vi "Pick&Place_ladder_shih_v8_toolcenter.vi"() -> ()   [LabVIEW 2016]
uses:
  WTF is this.ctl
  Classes/Controllers/I-O/Copy of NI-DAQ Folder/NI-DAQ.lvclass
  D:/INTT/V1/Classes/Controllers/I-O/Copy of I-O Folder/I-O.lvclass
  Classes/Controllers/Dispenser/Copy of Ultimus V2 Folder/Ultimus V2.lvclass
  <vilib>/Analysis/coordinate.llb/2D Cartesian Coordinate Rotation (Scalar).vi
  <vilib>/Utility/file.llb/Read Delimited Spreadsheet (DBL).vi
  <vilib>/Utility/file.llb/Write Delimited Spreadsheet (DBL).vi
  Classes/Controllers/Motion/Copy of Motion Folder/Motion.lvclass
  Classes/Controllers/Camera/Copy of Controller Folder/Controller.lvclass
  <vilib>/Analysis/NI_AALPro.lvlib
  Classes/Controllers/I-O/Copy of I-O Folder/I-O.lvclass
panel:
  out "file indicator":dbl[][](array[numeric])
  out "?":dbl[](array[numeric]) format="%#_8g"
  in  "offset":dbl[](array[numeric])=[0.0, 0.0, 0.0, 0.0] format="%#_8g"
  out "HDI center positions":dbl[][](array[numeric]) format="%#_8g"
  out "HDI center positions":dbl[][](array[numeric])=[[459.92445114002015, 980.2358762511564, 78.77350133595746, 0.0015214873297426886]] format="%#_8g"
  out "CT sum up":dbl[](array[numeric])
  in  "txt switch":bool
  in  "MPT offset":dbl[][](array[numeric])=[[0.0, 0.0, 0.0, 0.0], [0.0, 0.0, 0.0, 0.0]] format="%#_8g"
  out "CT HPoS":dbl[][](array[numeric]) format="%#_8g"
  out "chip distance by OGP":dbl format="%#_8g"
  out "displacement":dbl[](array[numeric])
  out "gantry position test":dbl[](array[numeric])
  out "gantry target position":dbl[](array[numeric])
  out "chip distance by gantry":dbl format="%#_8g"
  out "after SL":dbl[](array[numeric]) format="%#_8g"
  out "after SR":dbl[](array[numeric]) format="%#_8g"
  out "after NL":dbl[](array[numeric]) format="%#_8g"
  out "S chip":dbl[](array[numeric]) format="%#_8g"
  out "N chip":dbl[](array[numeric]) format="%#_8g"
  in  "?":path=path "C:/Users/PAGANIS/Desktop/shih cheng wei/OGP/test1-2.txt"
  out "bless from OGP !!! Center of  stave":dbl[](array[numeric])
  out "bless from OGP !! measured stave size":dbl[](array[numeric])
  in  "Bless from OGP":bool
  out "FROM Detail !!! Center of module on stave":dbl[](array[numeric])
  out "FROM Detail !! measured stave size":dbl[](array[numeric])
  in  "Align Stave in detail":bool
  in  "check height?":bool
  in  "Uttimus presssure":i64=10
  out "Status":bool
  out "measured HDI top-left position":dbl[][](array[numeric])
  in  "HDI vacuum channel":i32=18
  in  "vacuum":bool=TRUE
  in  "HDI vacuum":bool
  out "measured stave size":dbl[](array[numeric])
  out "Stave mark":dbl[][](array[numeric])
  out "Center of module on stave":dbl[](array[numeric])
  out "Measured HDI size":dbl[][](array[numeric])
  out "MPT positions on stave":T1[][](array[typedef])
  in  "Default Stave dimension":dbl[](array[numeric])=[34.0, 472.0, -0.335295, -0.000320234]
  in  "Default Stave upper left mark":dbl[](array[numeric])=[584.376, 675.576, 70.9882, 0.000840064]
  out "Needle parking position":dbl[](array[numeric])
  in  "Uppler / Lower Stave":bool=TRUE
  out "Gantry current position":dbl[](array[numeric])
  in  "READ Position":bool
  in  "Needle Height Compenstation\n(glue gap)":dbl=0.33
  in  "Needle Alignment":bool
  in  "Parking position":dbl[](array[numeric])=[625.0, 625.0, 0.0, 0.01]
  in  "GOTO":bool
  in  "Default Pickup Tool Position":dbl[][](array[numeric])=[[152.226, 682.729, 36.8129, -0.0151898], [700.0, 800.0, 20.0, 0.01]]
  in  "deposit glue module":i32=1
  in  "Default HDI alignment \nmark position":dbl[](array[numeric])=[448.322, 976.582, 74.9872, 0.000191129]
  in  "Default HDI size":dbl[](array[numeric])=[24.2437, 231.446, -0.099339, 0.000191129]
  out "# of tasks excuted":i32
  out "PickupTool \nCenterPosition":dbl[](array[numeric]) format="%#_8g"
  in  "Inititalize":bool
  in  "Pick and place":bool
  in  "Deposit Glue":bool
  in  "Measure Pickup Tools":bool
  in  "Align Stave":bool
  out "default module position on stave":dbl[][](array[numeric])
  in  "Stop":bool
  in  "Measure HDI":bool
  # "Ladder Assembly"
  # "To switch the north/south\ntxt file \nswitch \noffset\nmodule pick up tool\nmodule direction"
  # "Upper\nmodule"
  # "Lower\nmodule"
  # "Sensor 0.32 -> 200 micron glue thickness\nChips 0.37-> 140 micron glue thickness"
  # "ACTIONS"
  # "theta had *-1"
  # "Pick up tool and needle"
  # "Module infomation"
  # "Pick and Place"
  # "CT"
  # "+"
  # "+"
  # "="
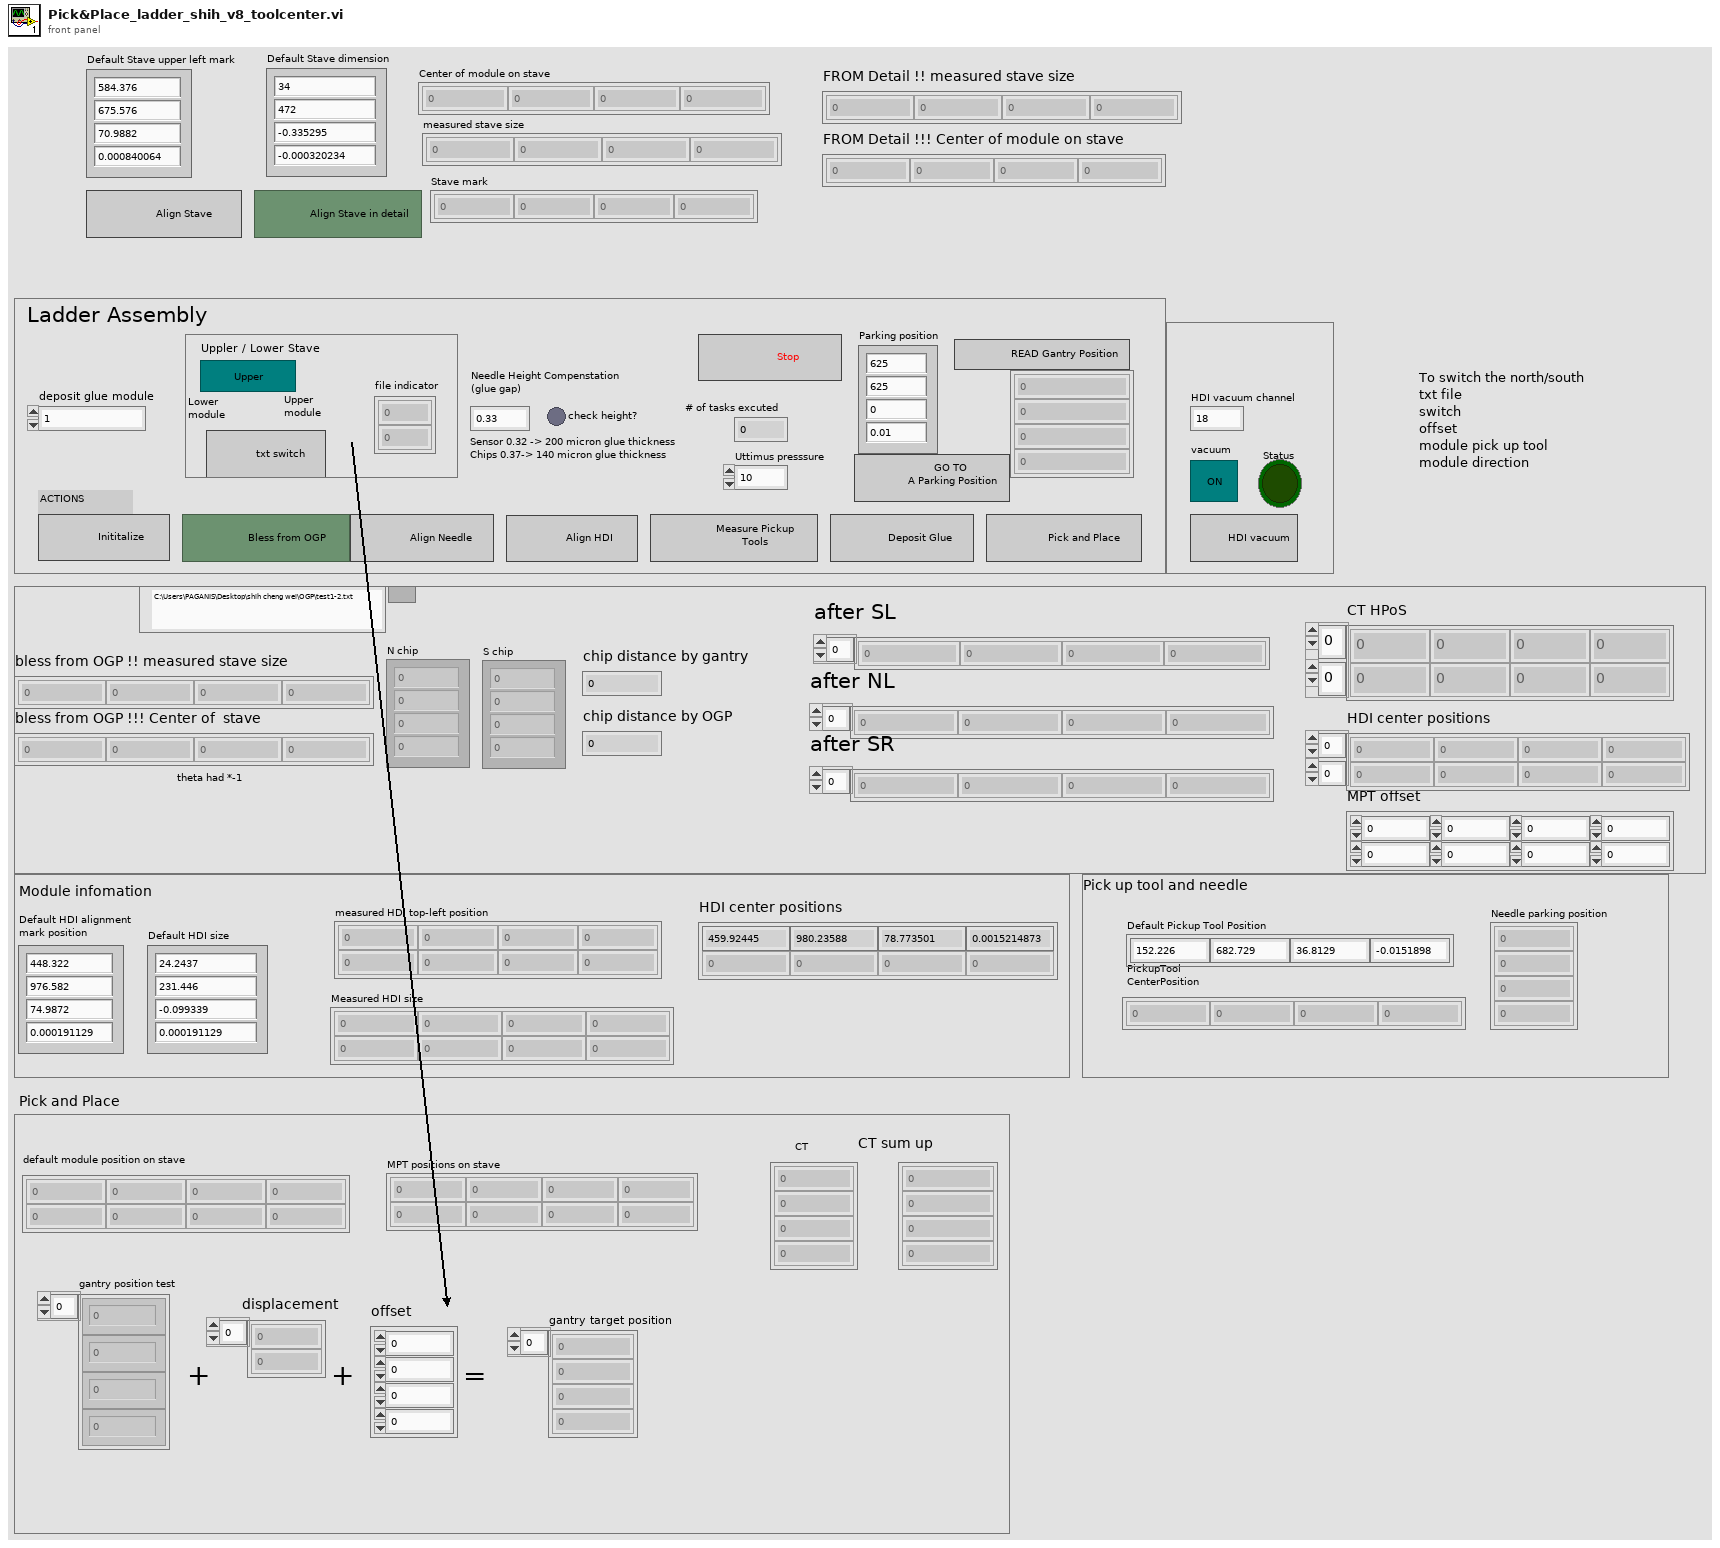
[diagram p1: front panel]
types:
  T1 = typedef "WTF is this.ctl" = dbl
  T2 = typedef "Controller.lvclass/Controllers.ctl" = cluster{"Copy of Motion.lvclass":refnum<class "Motion.lvclass">, "Copy of I-O.lvclass":refnum<class "I-O.lvclass">, "Copy of Dispenser.lvclass":refnum<class "Dispenser.lvclass">}
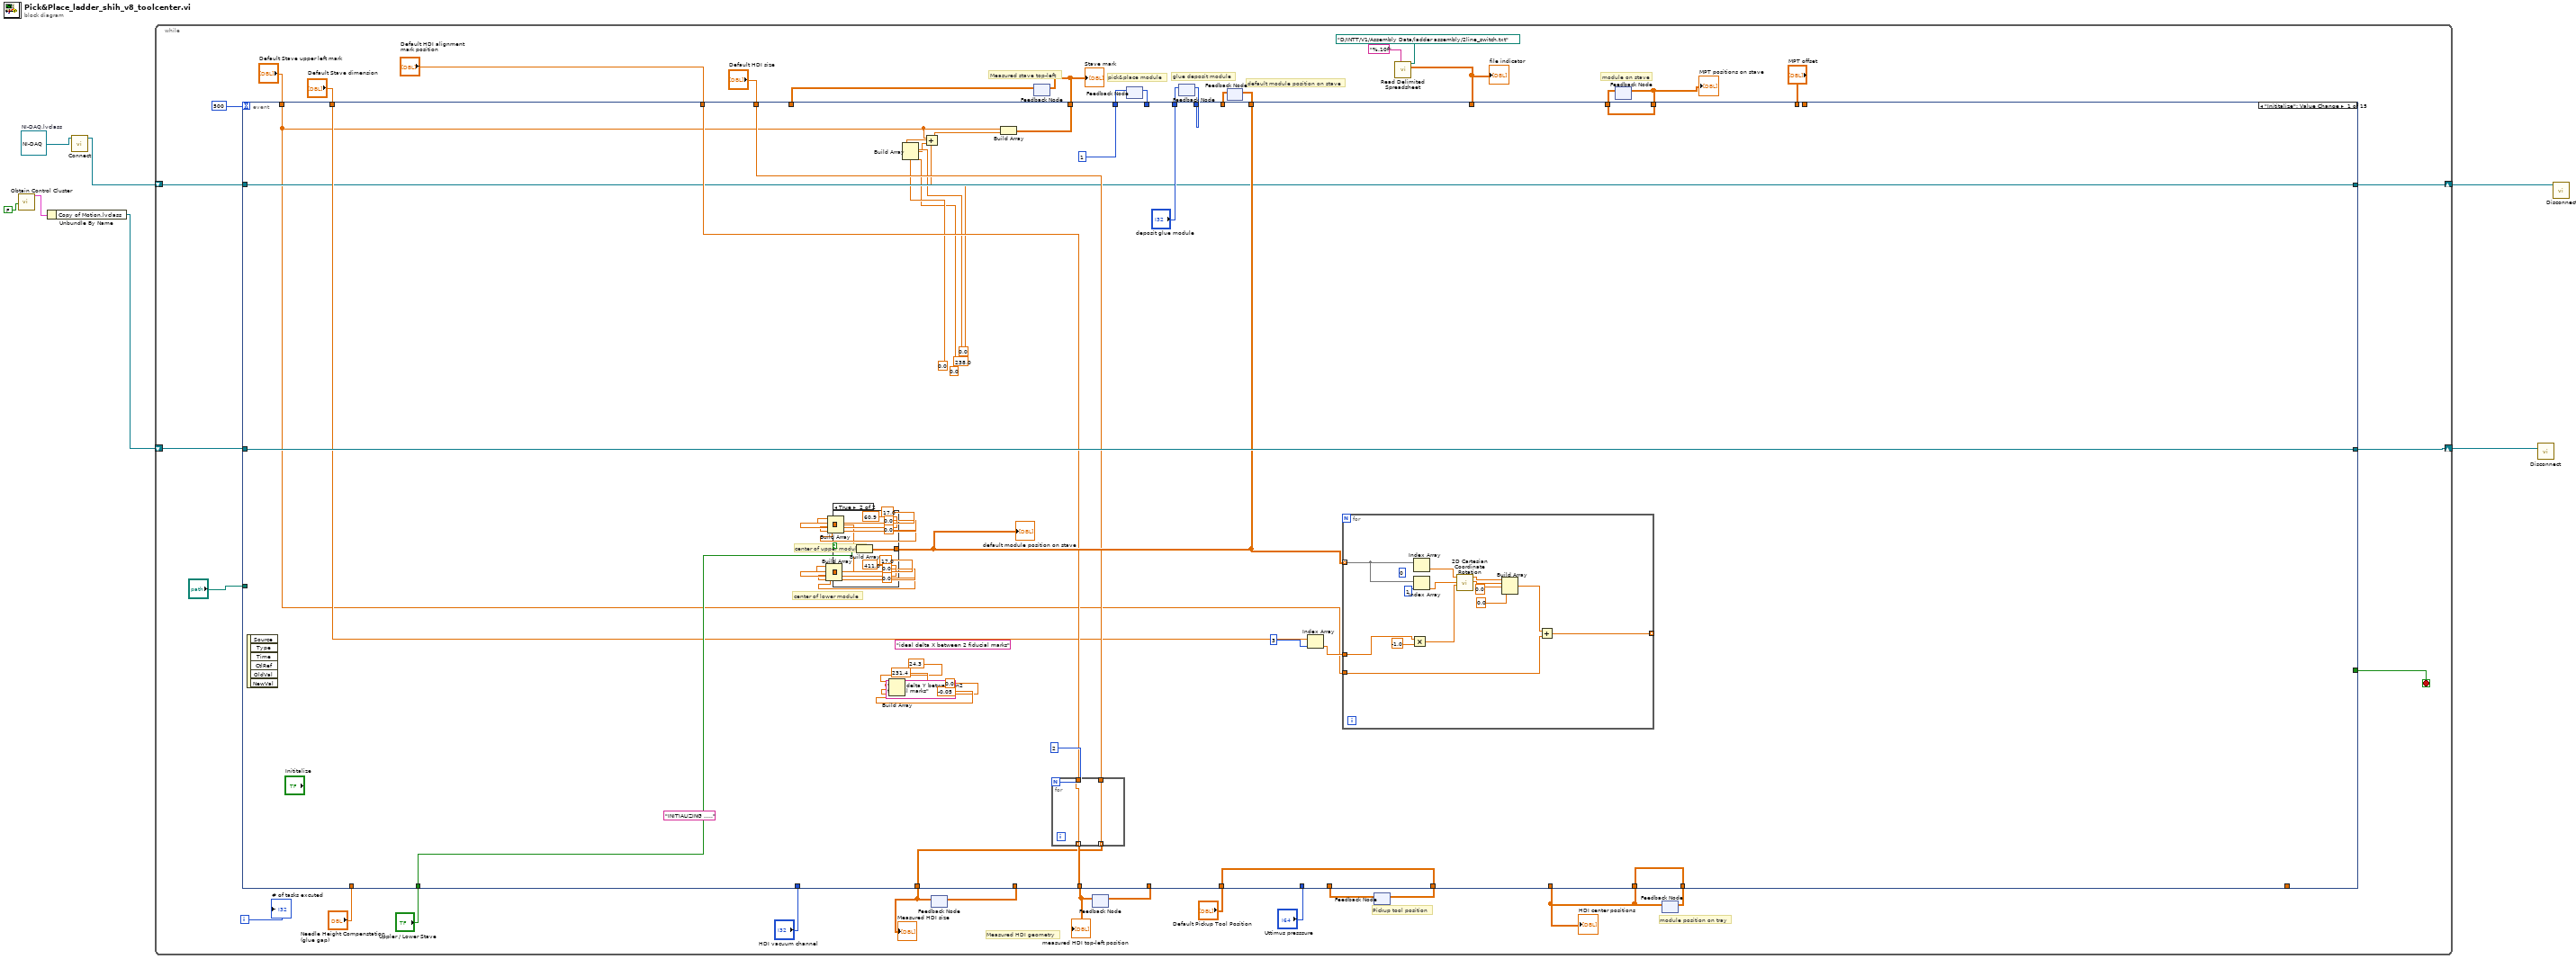
[diagram p0: block diagram]
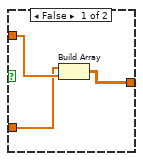
[diagram p2: hidden frame]
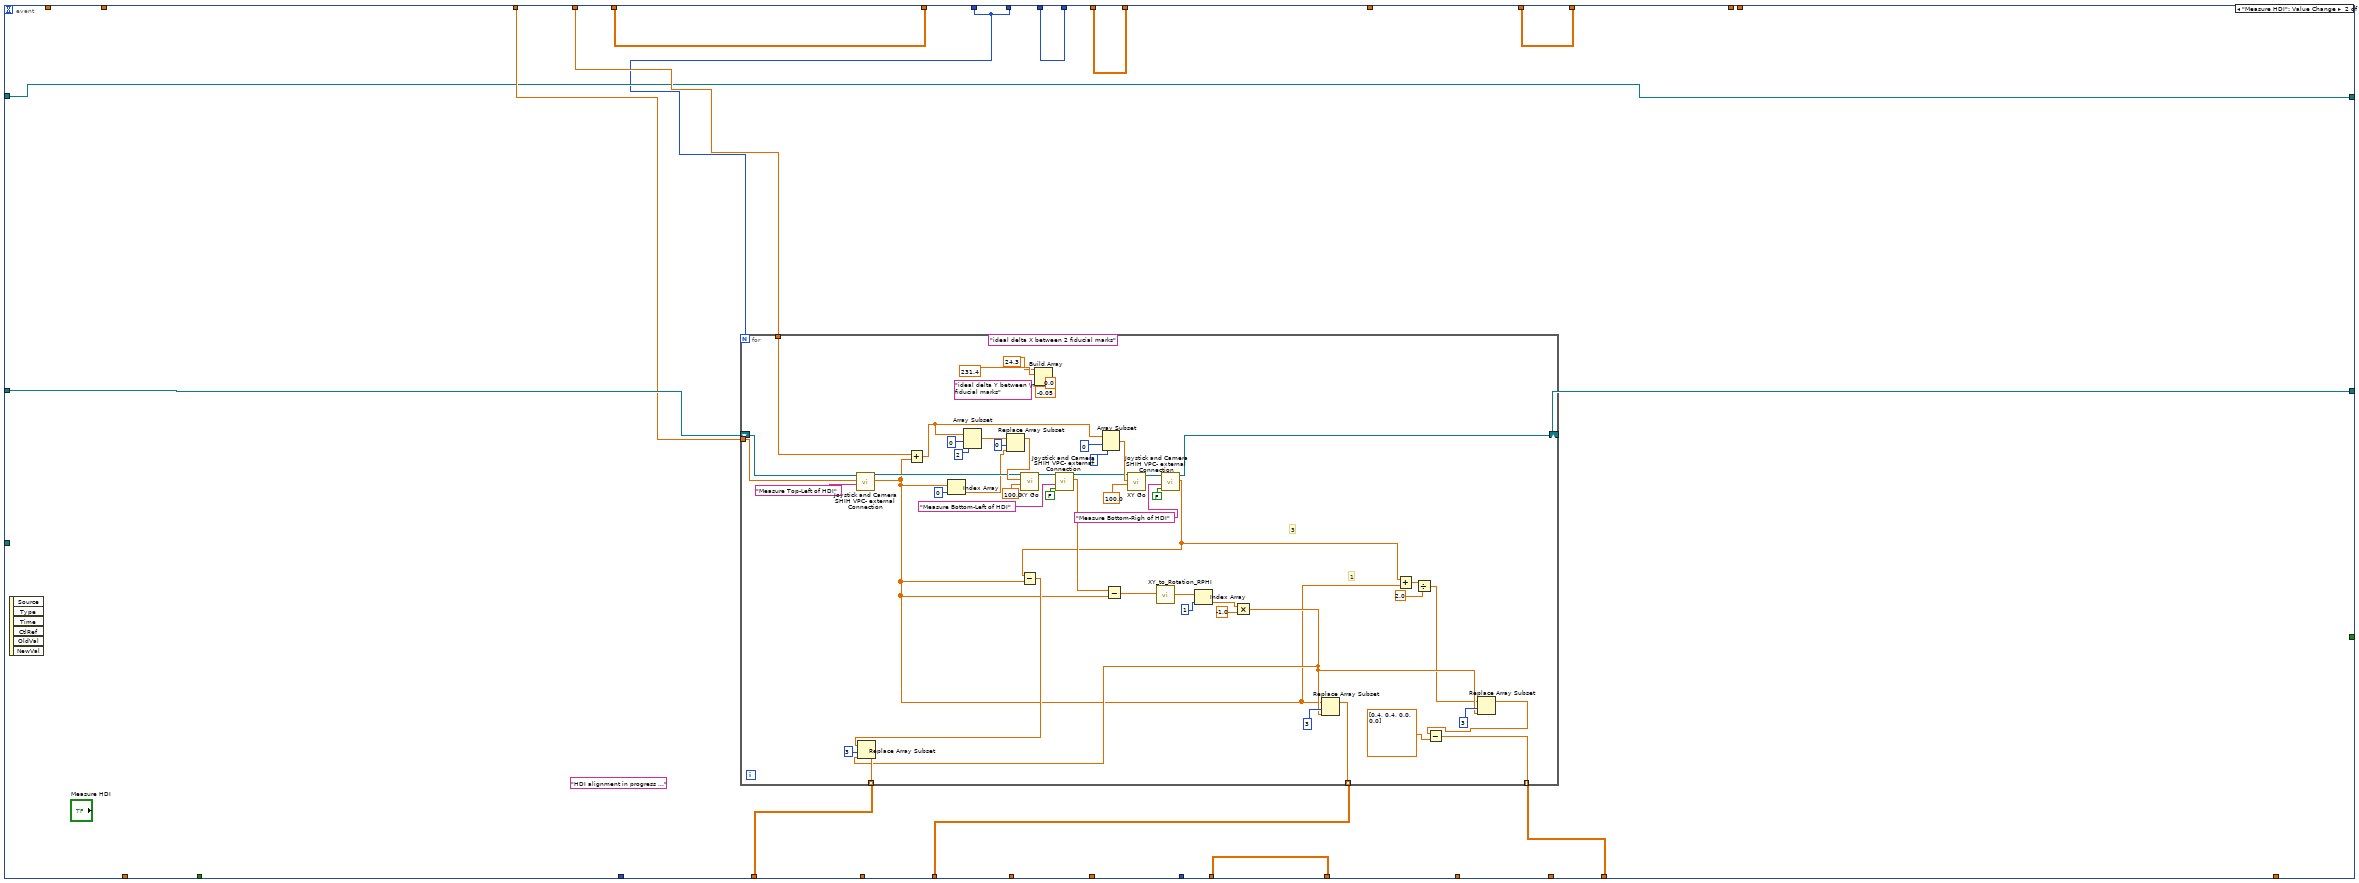
[diagram p3: hidden frame]
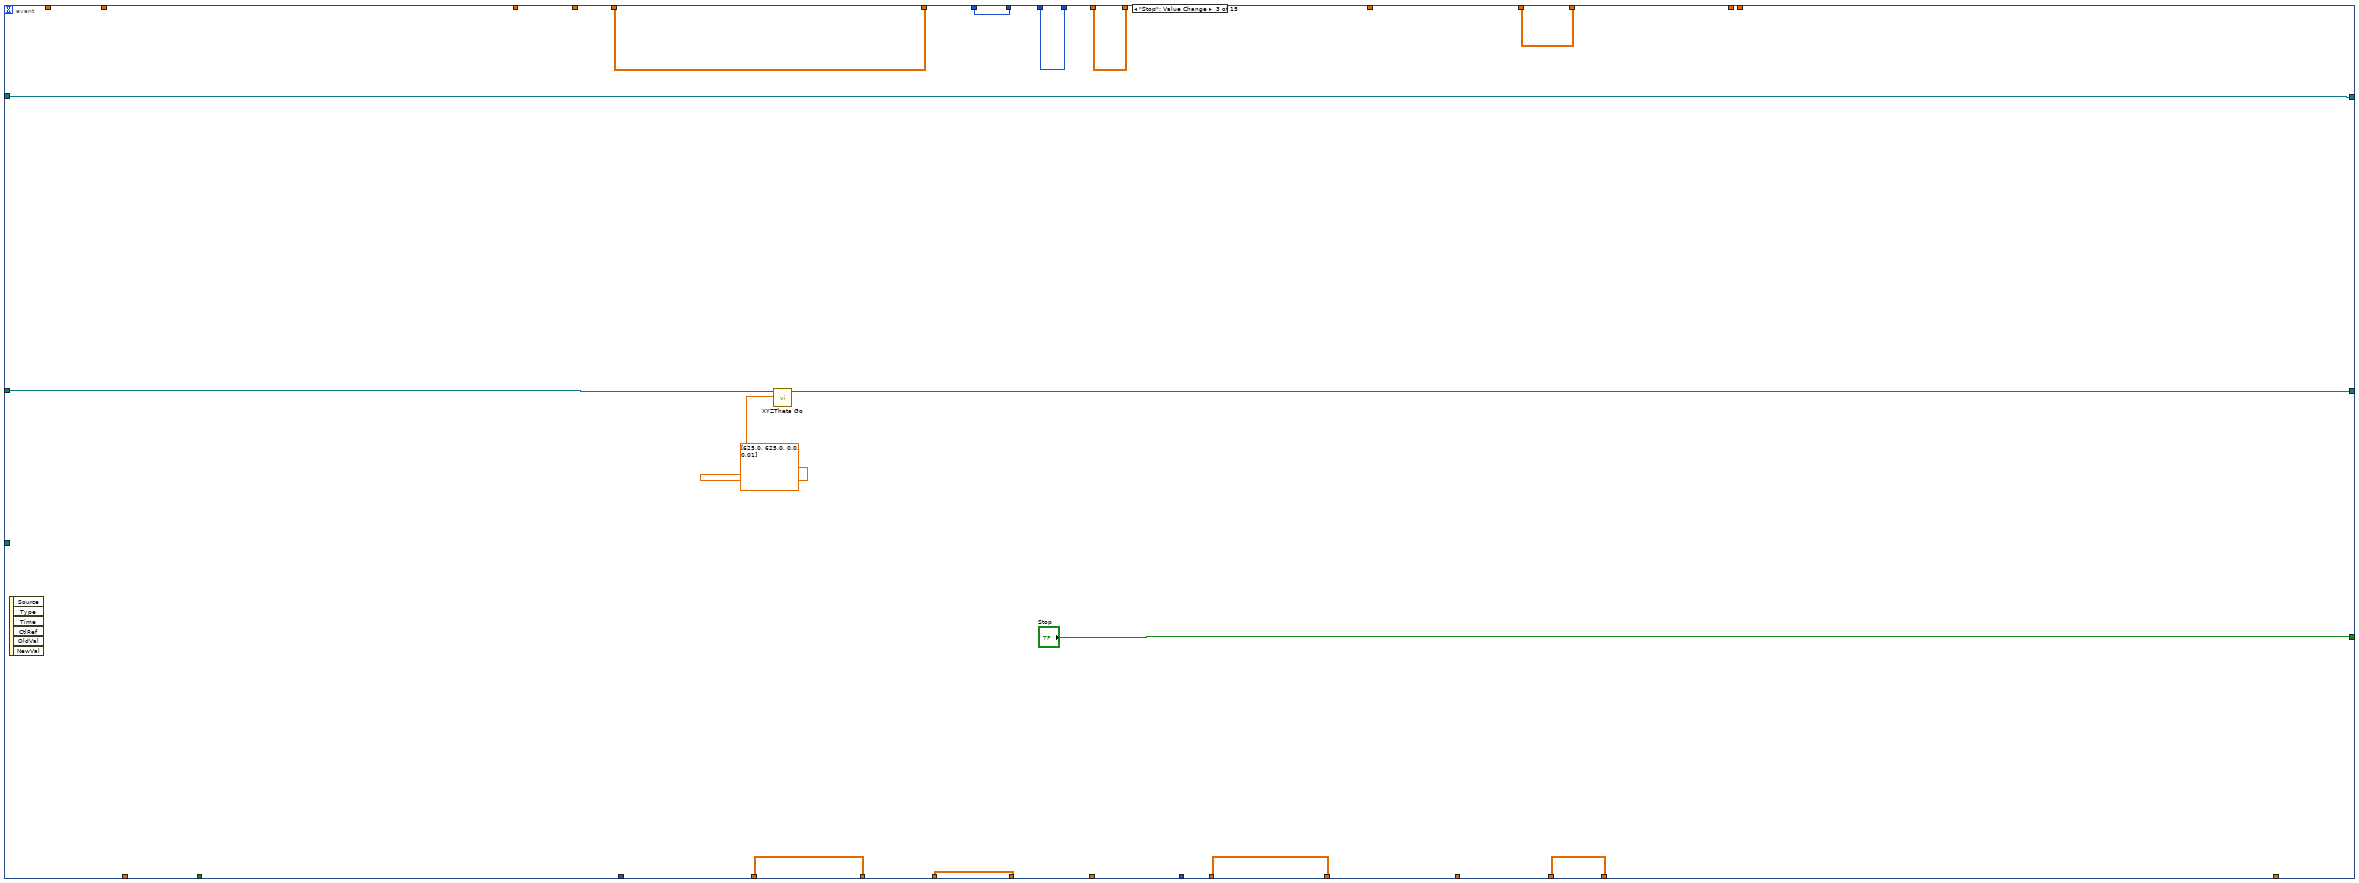
[diagram p4: hidden frame]
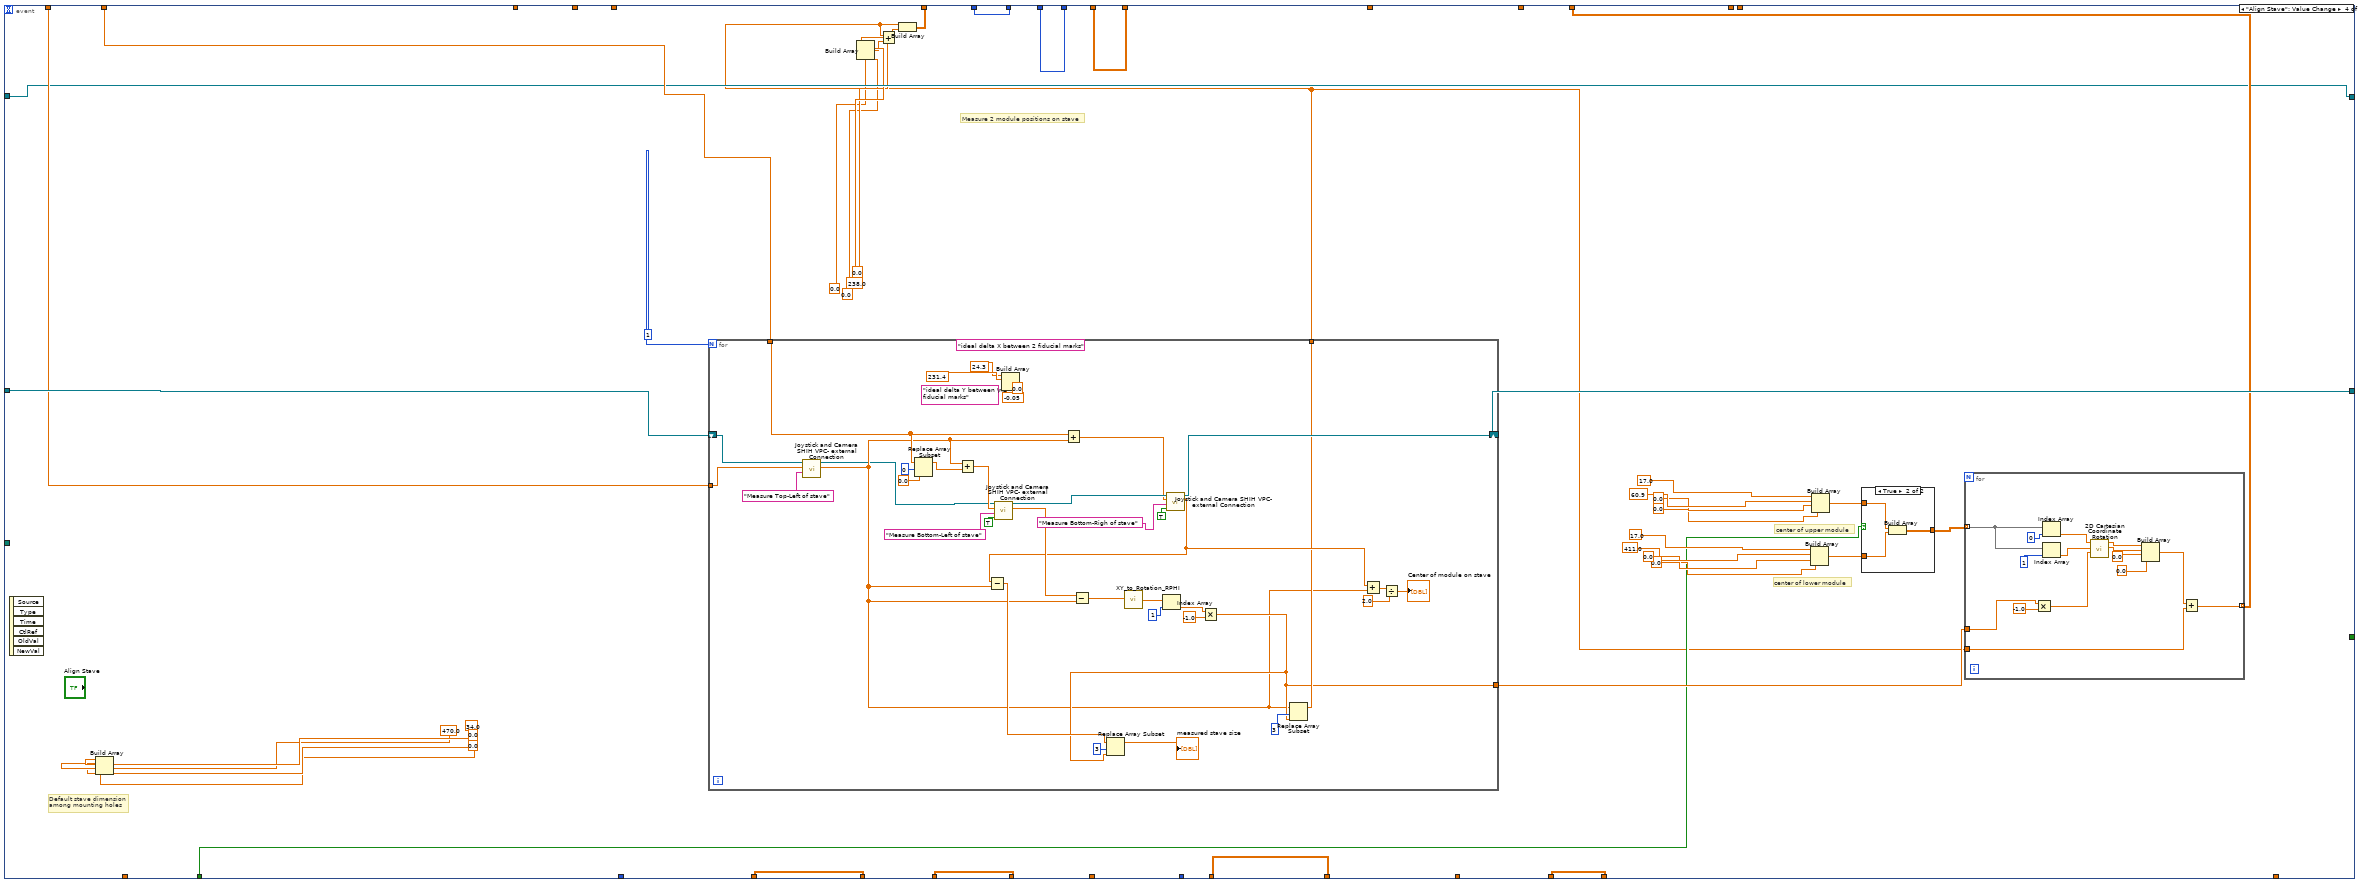
[diagram p5: hidden frame]
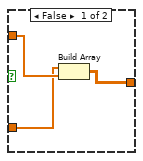
[diagram p6: hidden frame]
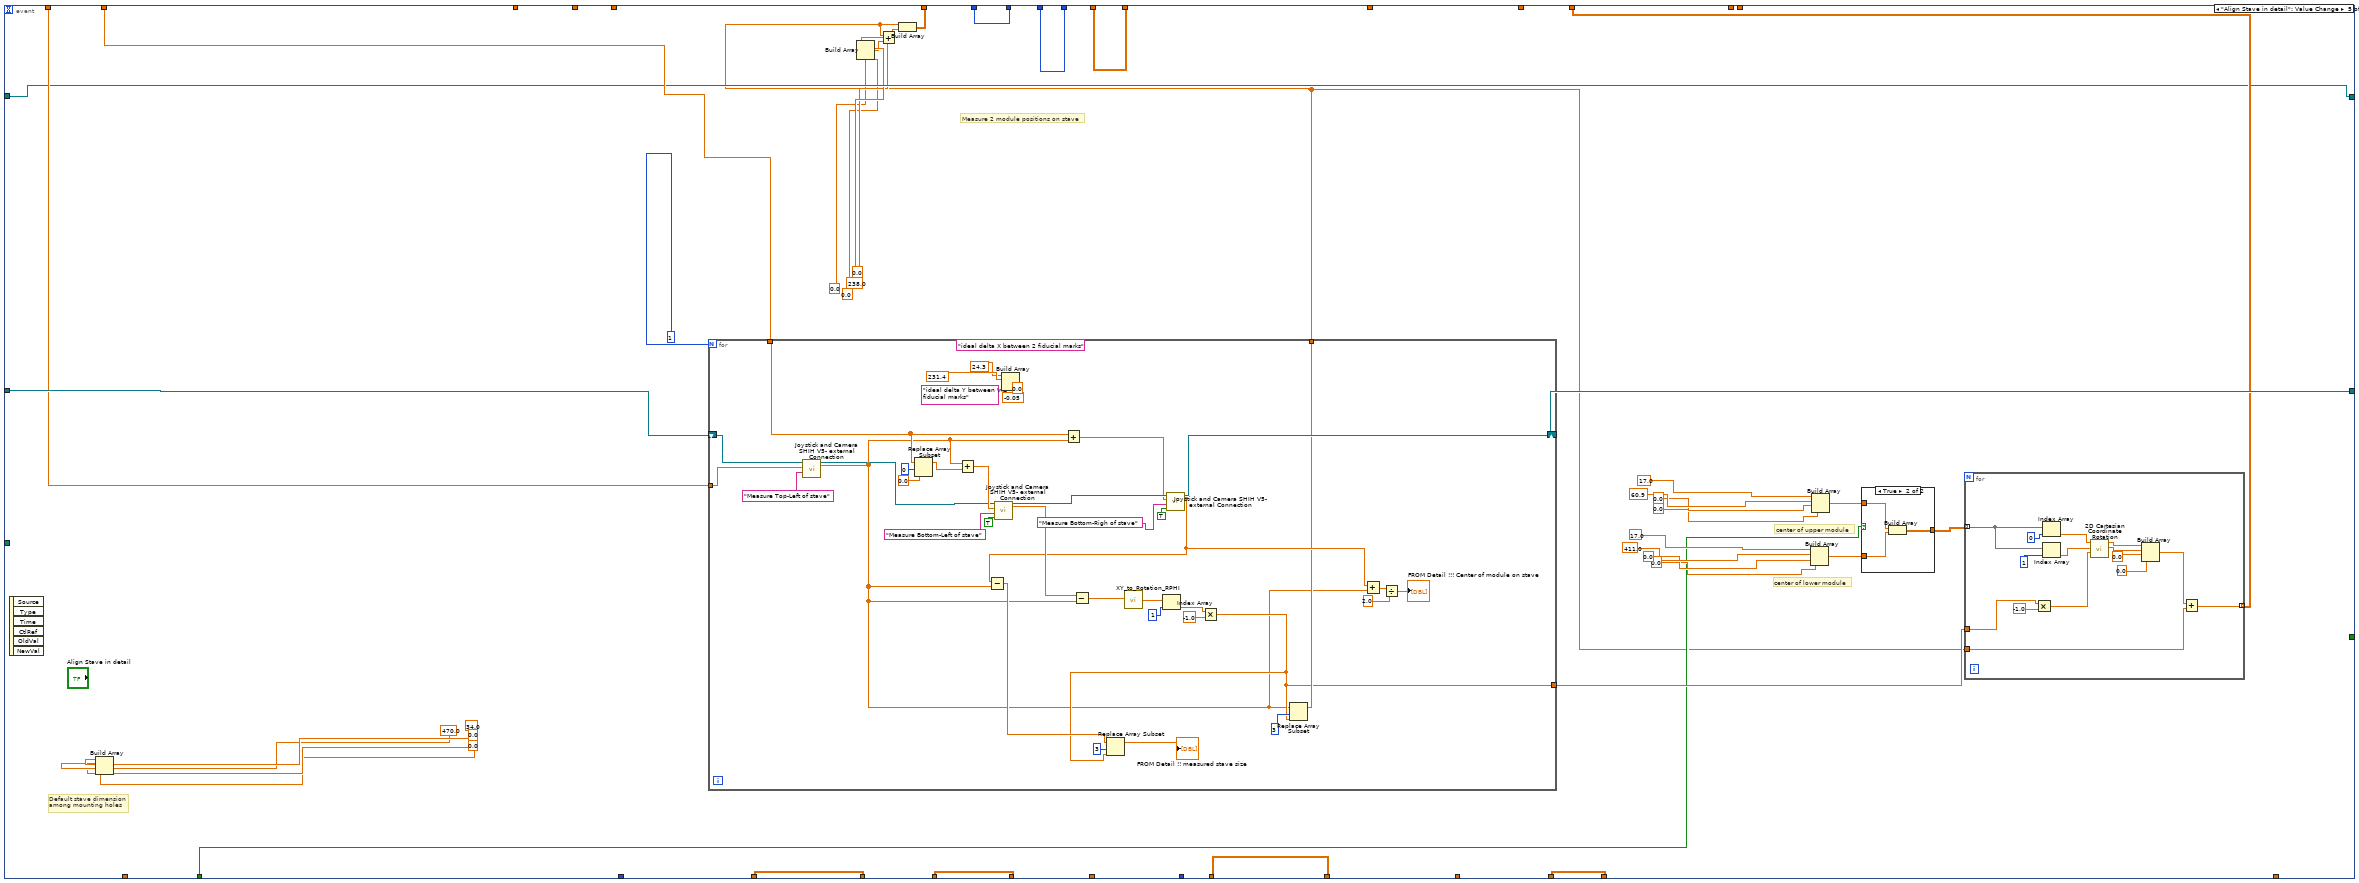
[diagram p7: hidden frame]
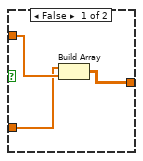
[diagram p8: hidden frame]
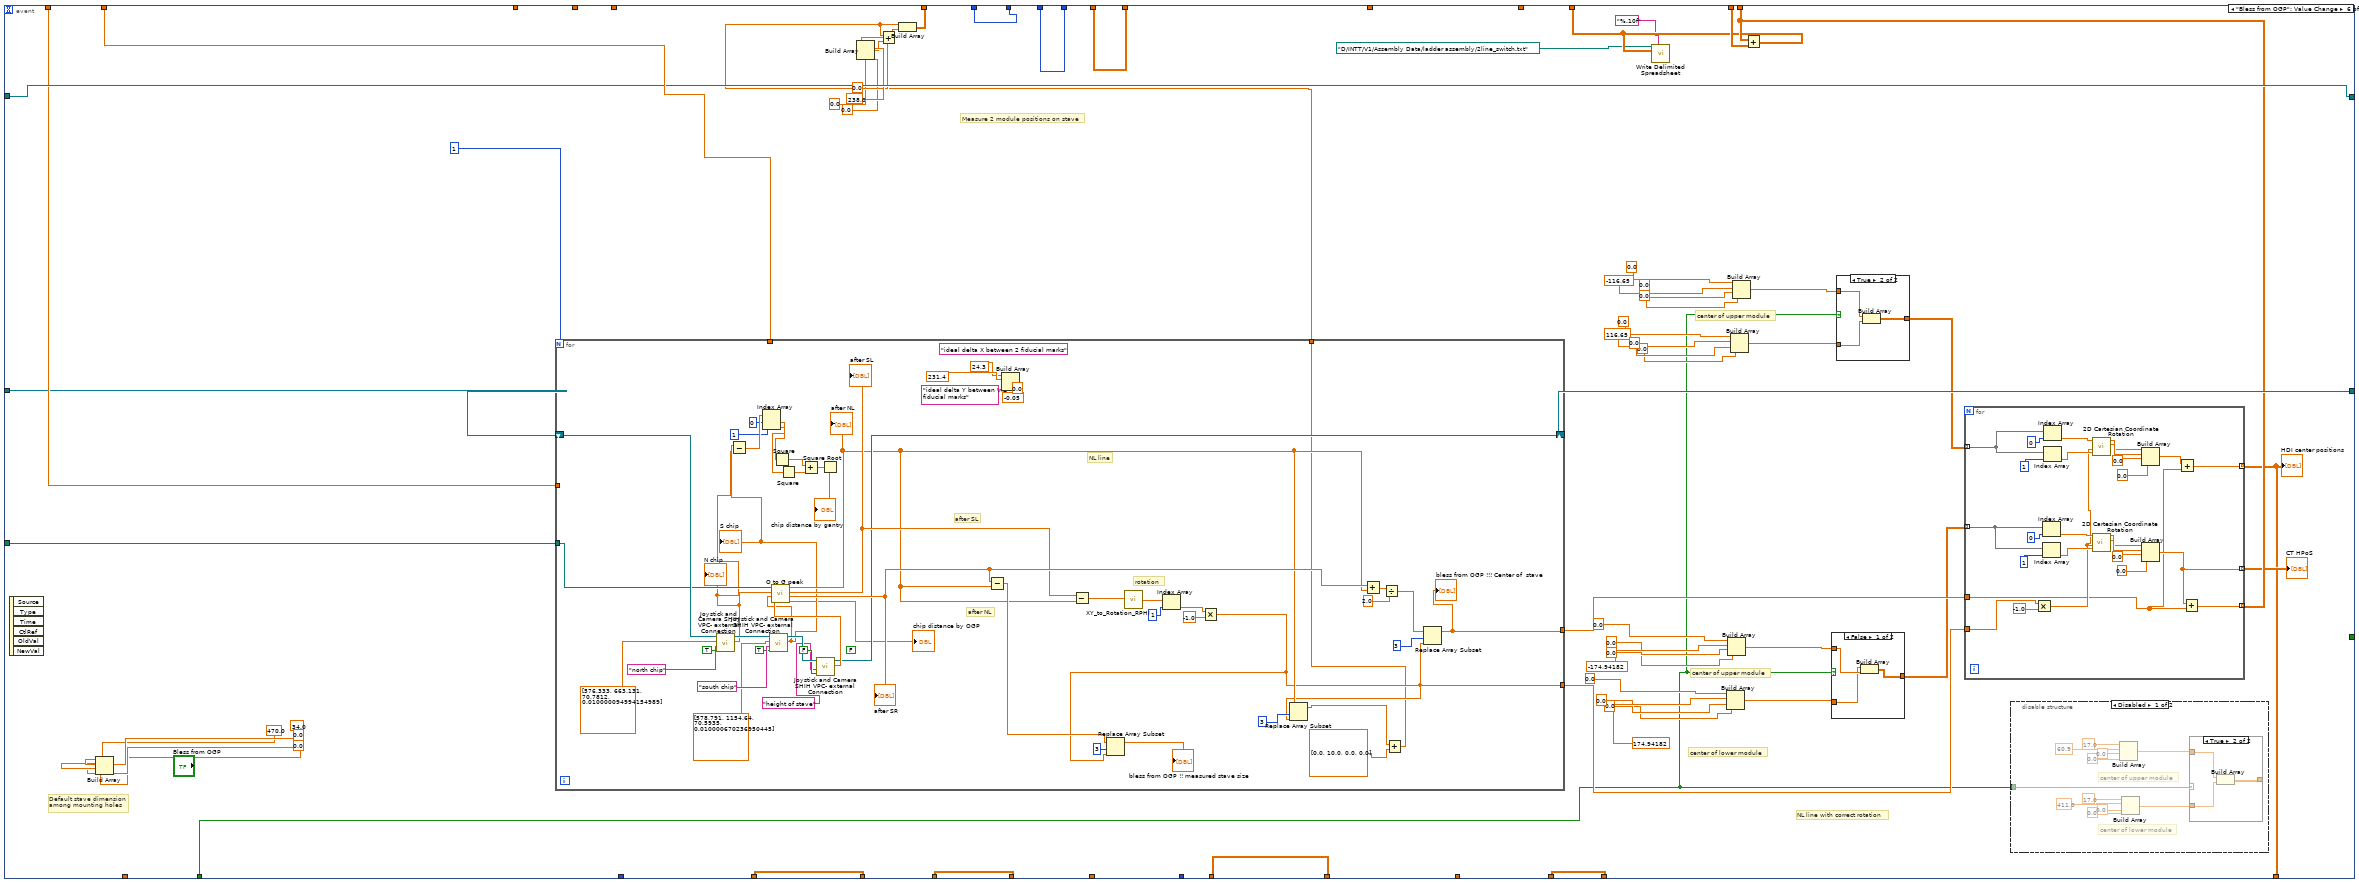
[diagram p9: hidden frame]
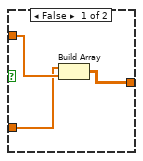
[diagram p10: hidden frame]
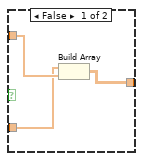
[diagram p11: hidden frame]
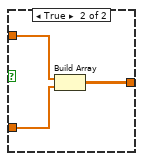
[diagram p13: hidden frame]
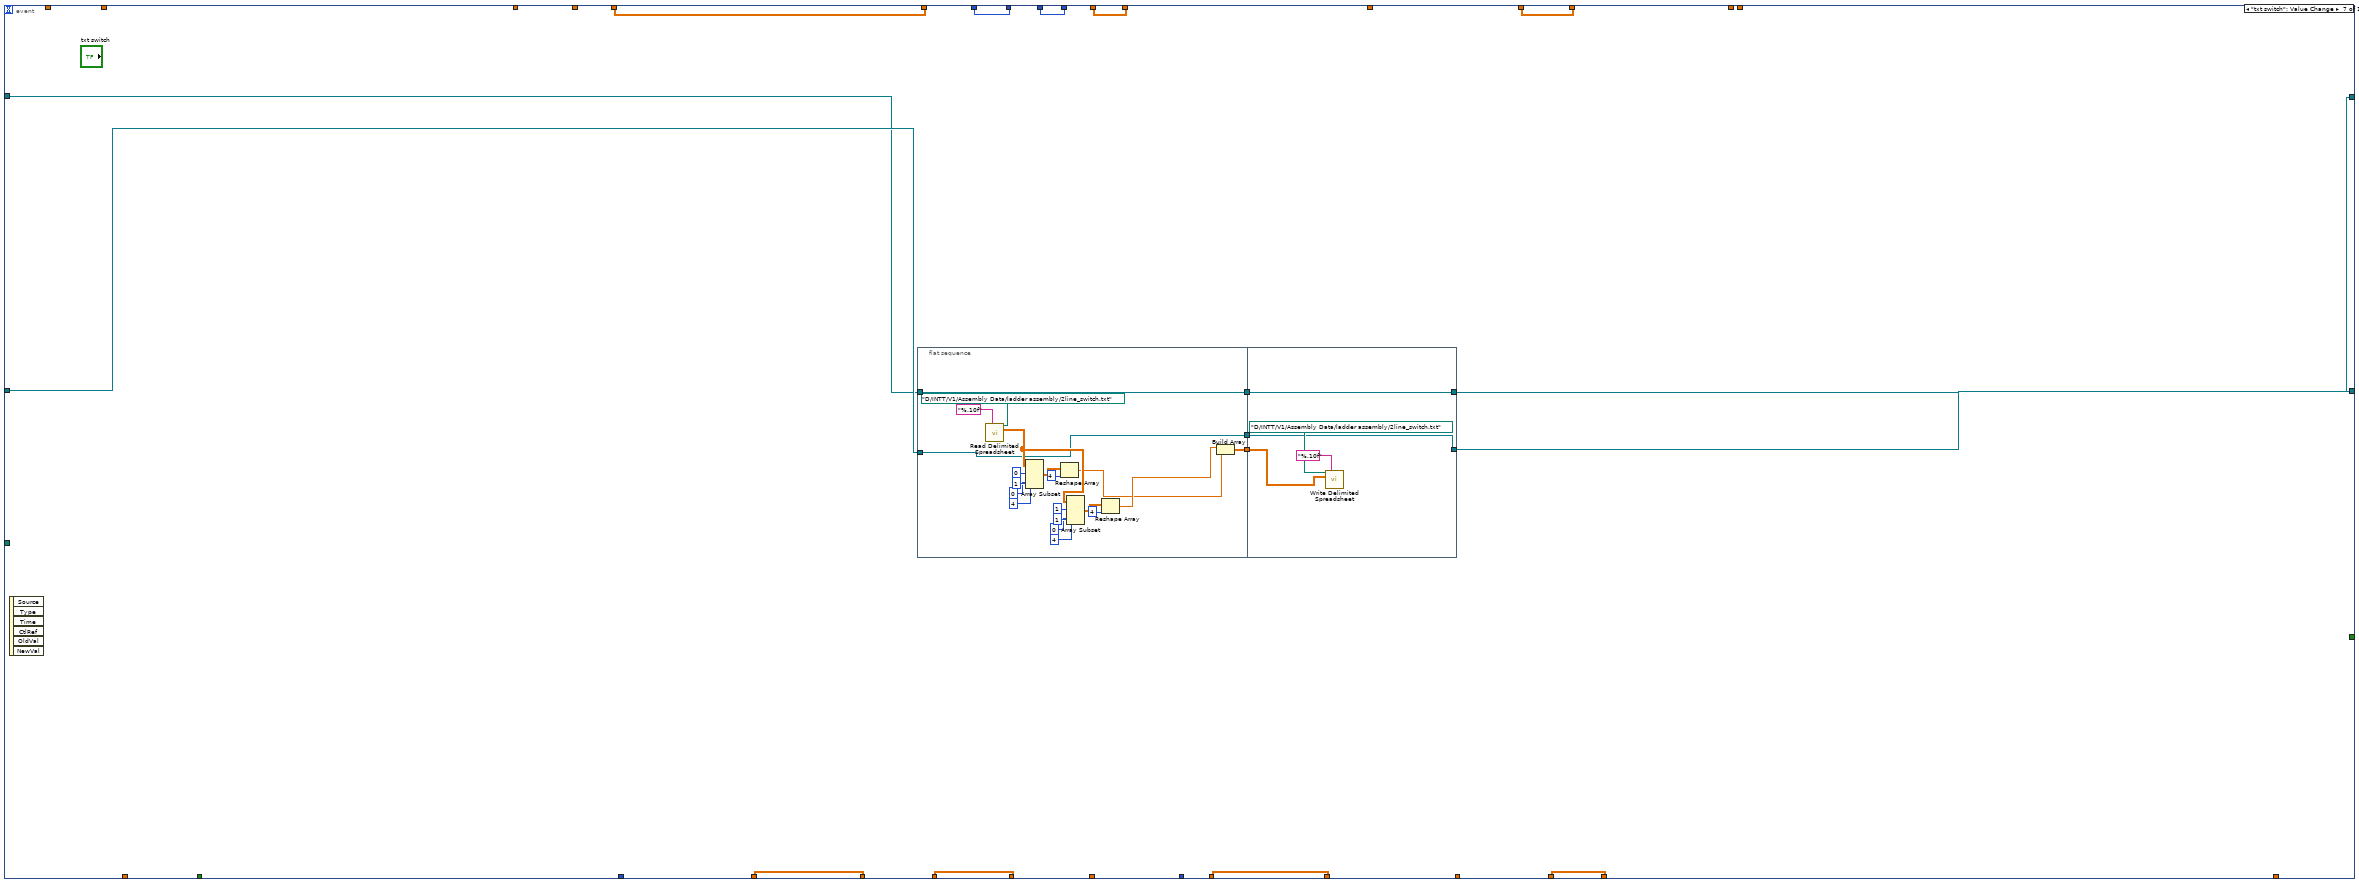
[diagram p14: hidden frame]
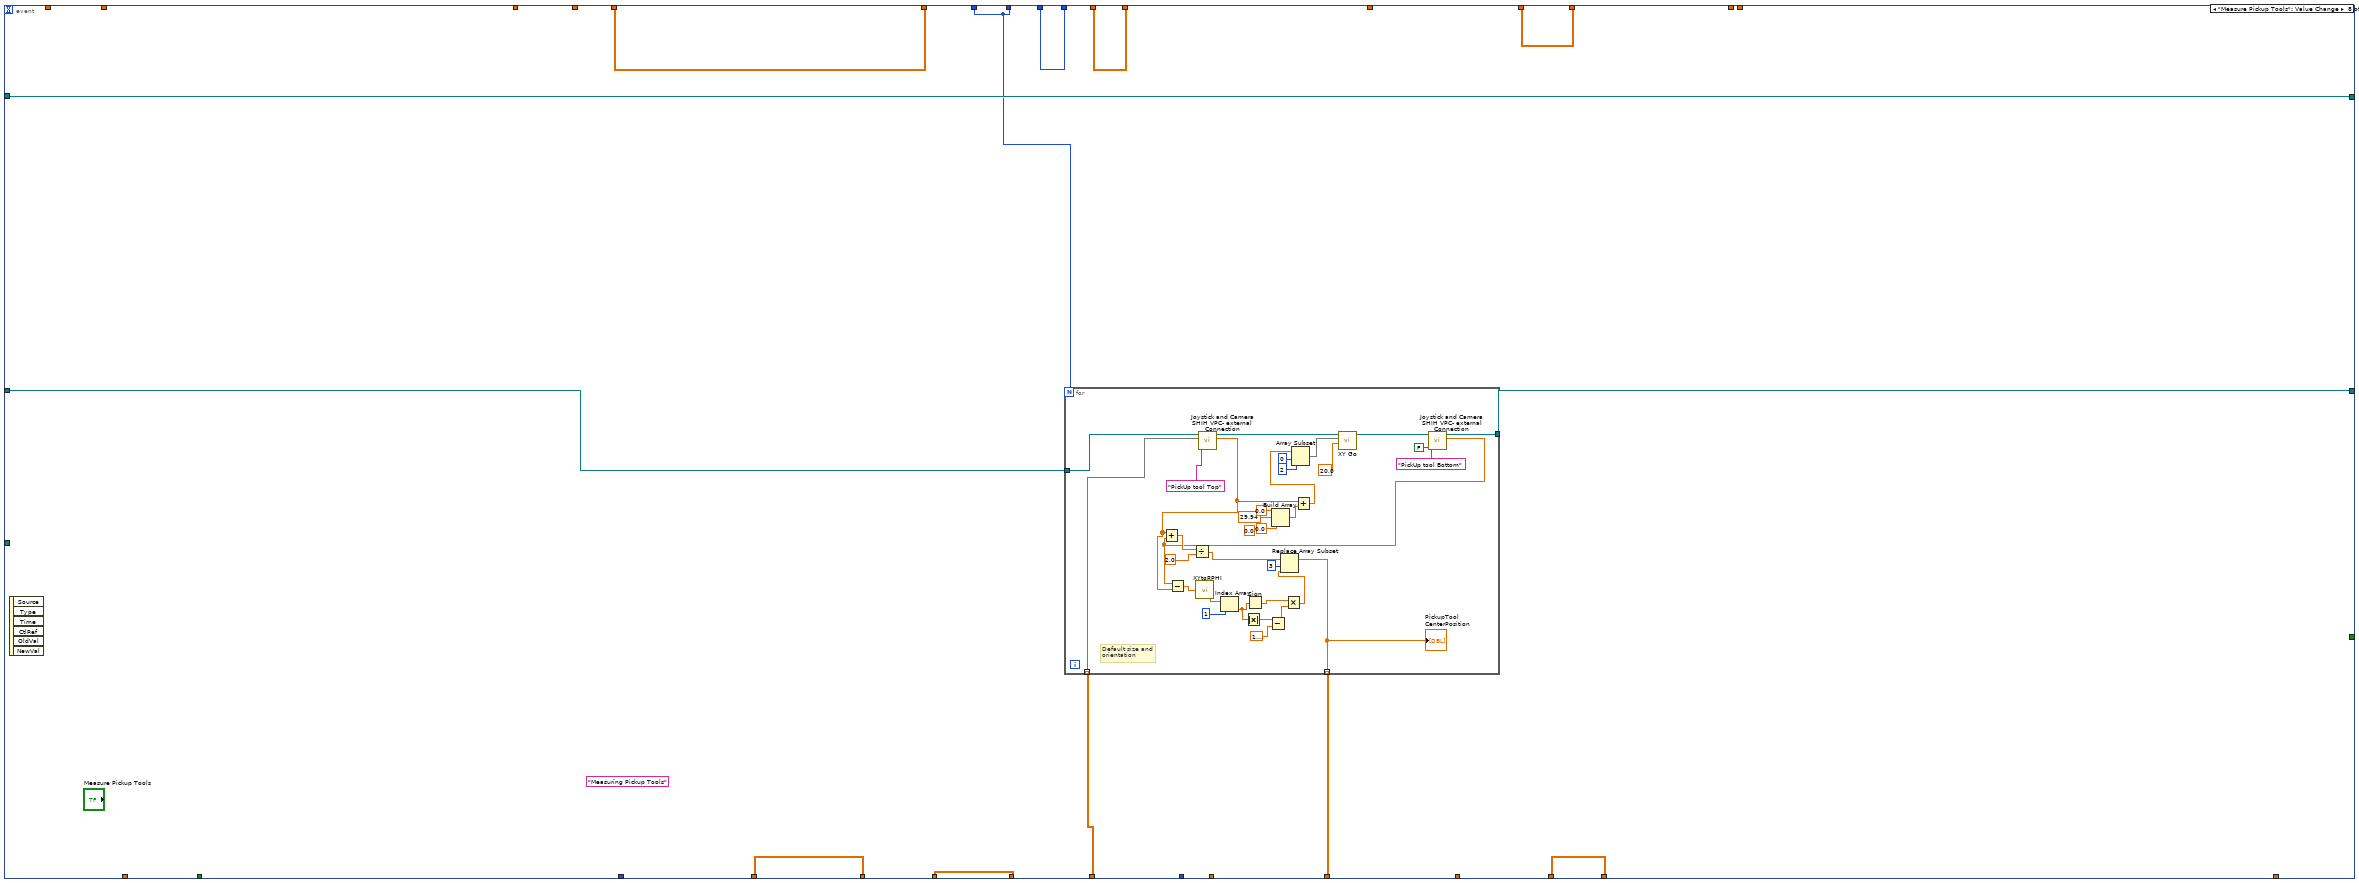
[diagram p15: hidden frame]
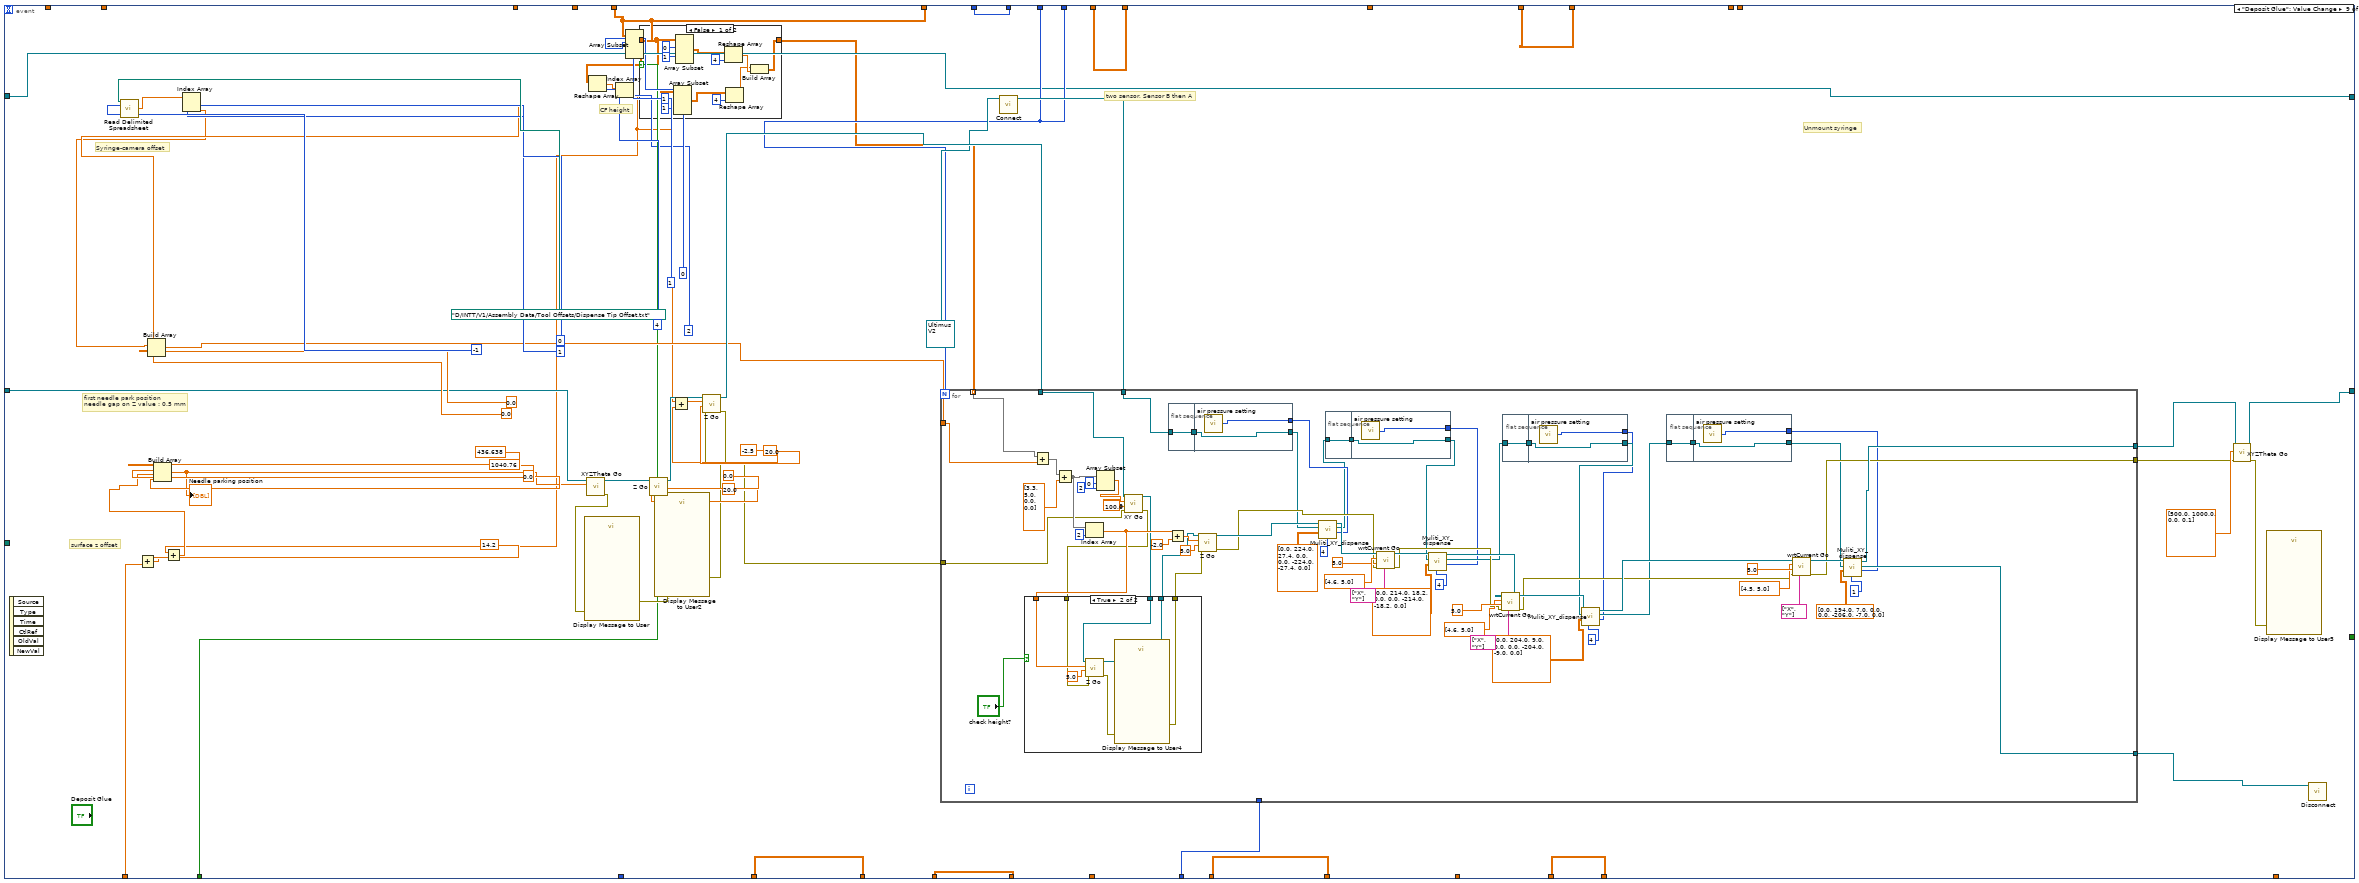
[diagram p16: hidden frame]
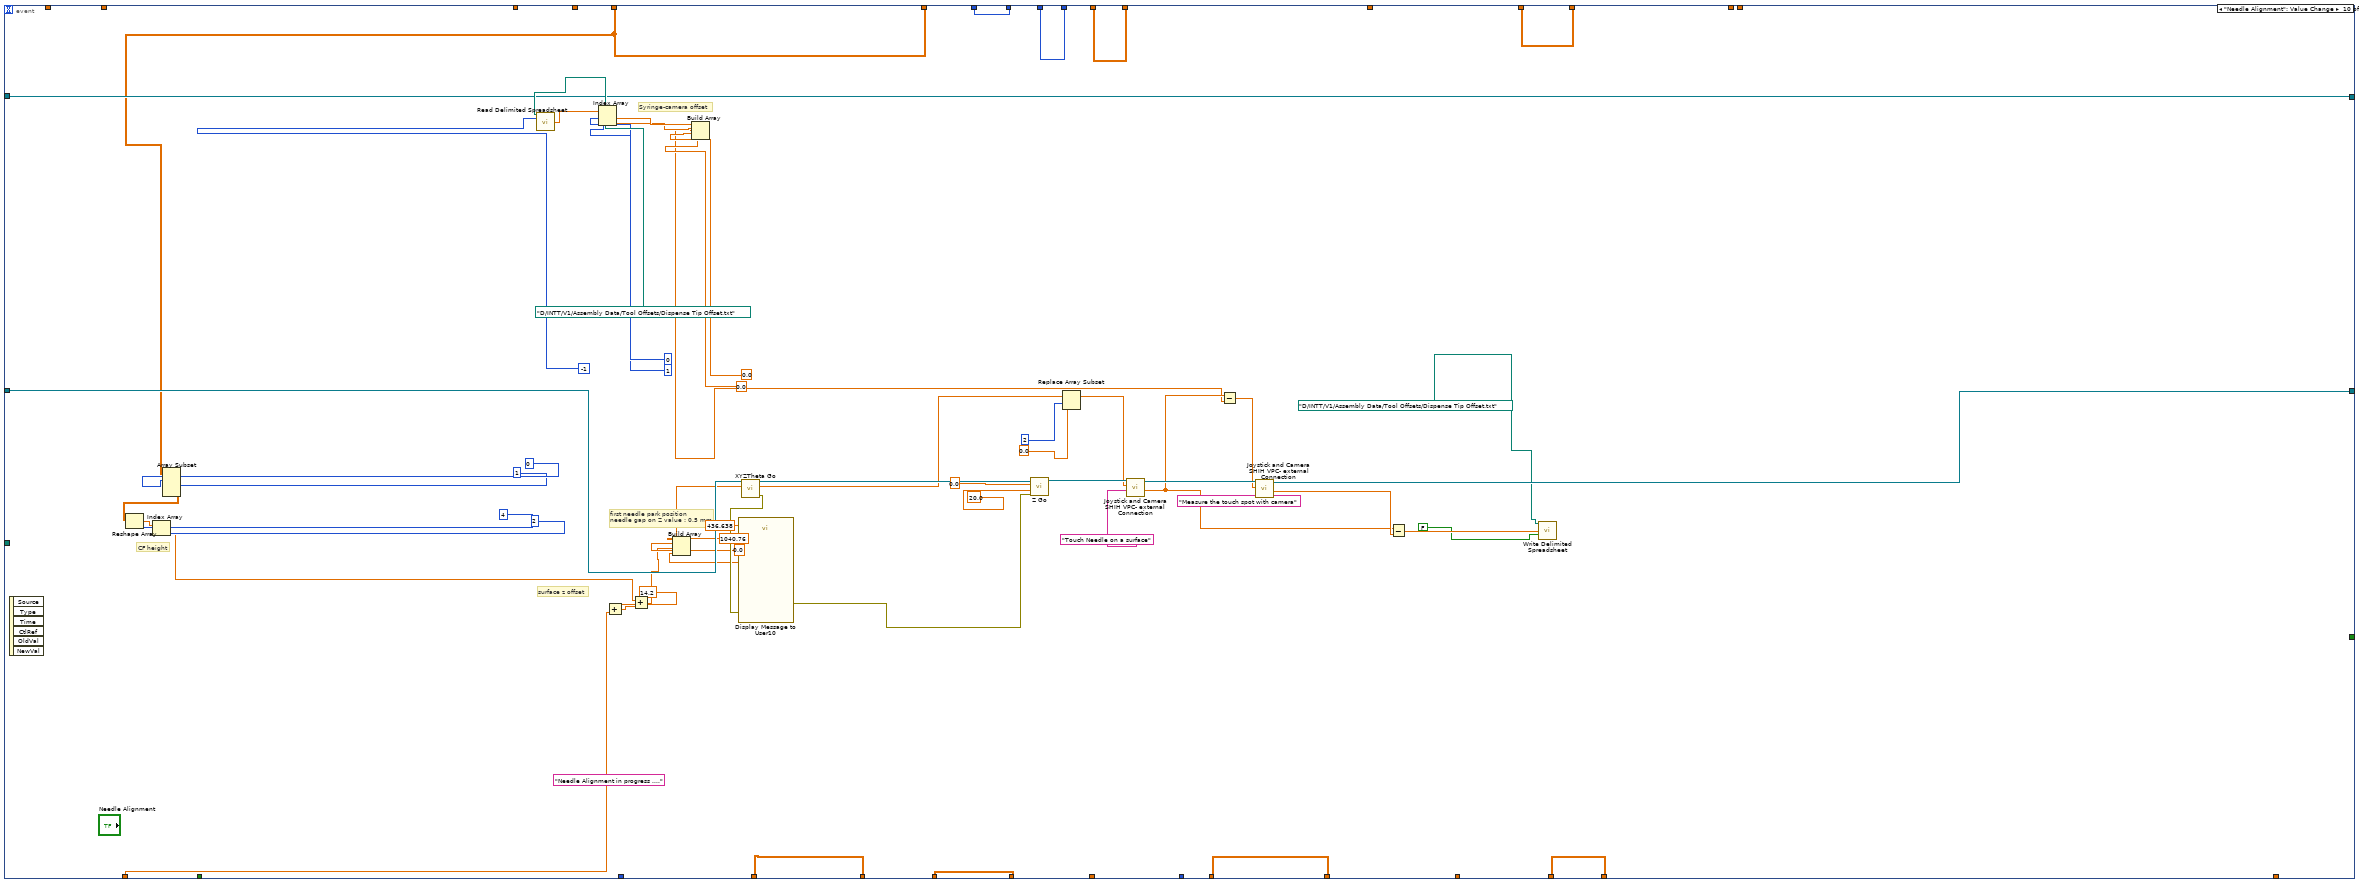
[diagram p19: hidden frame]
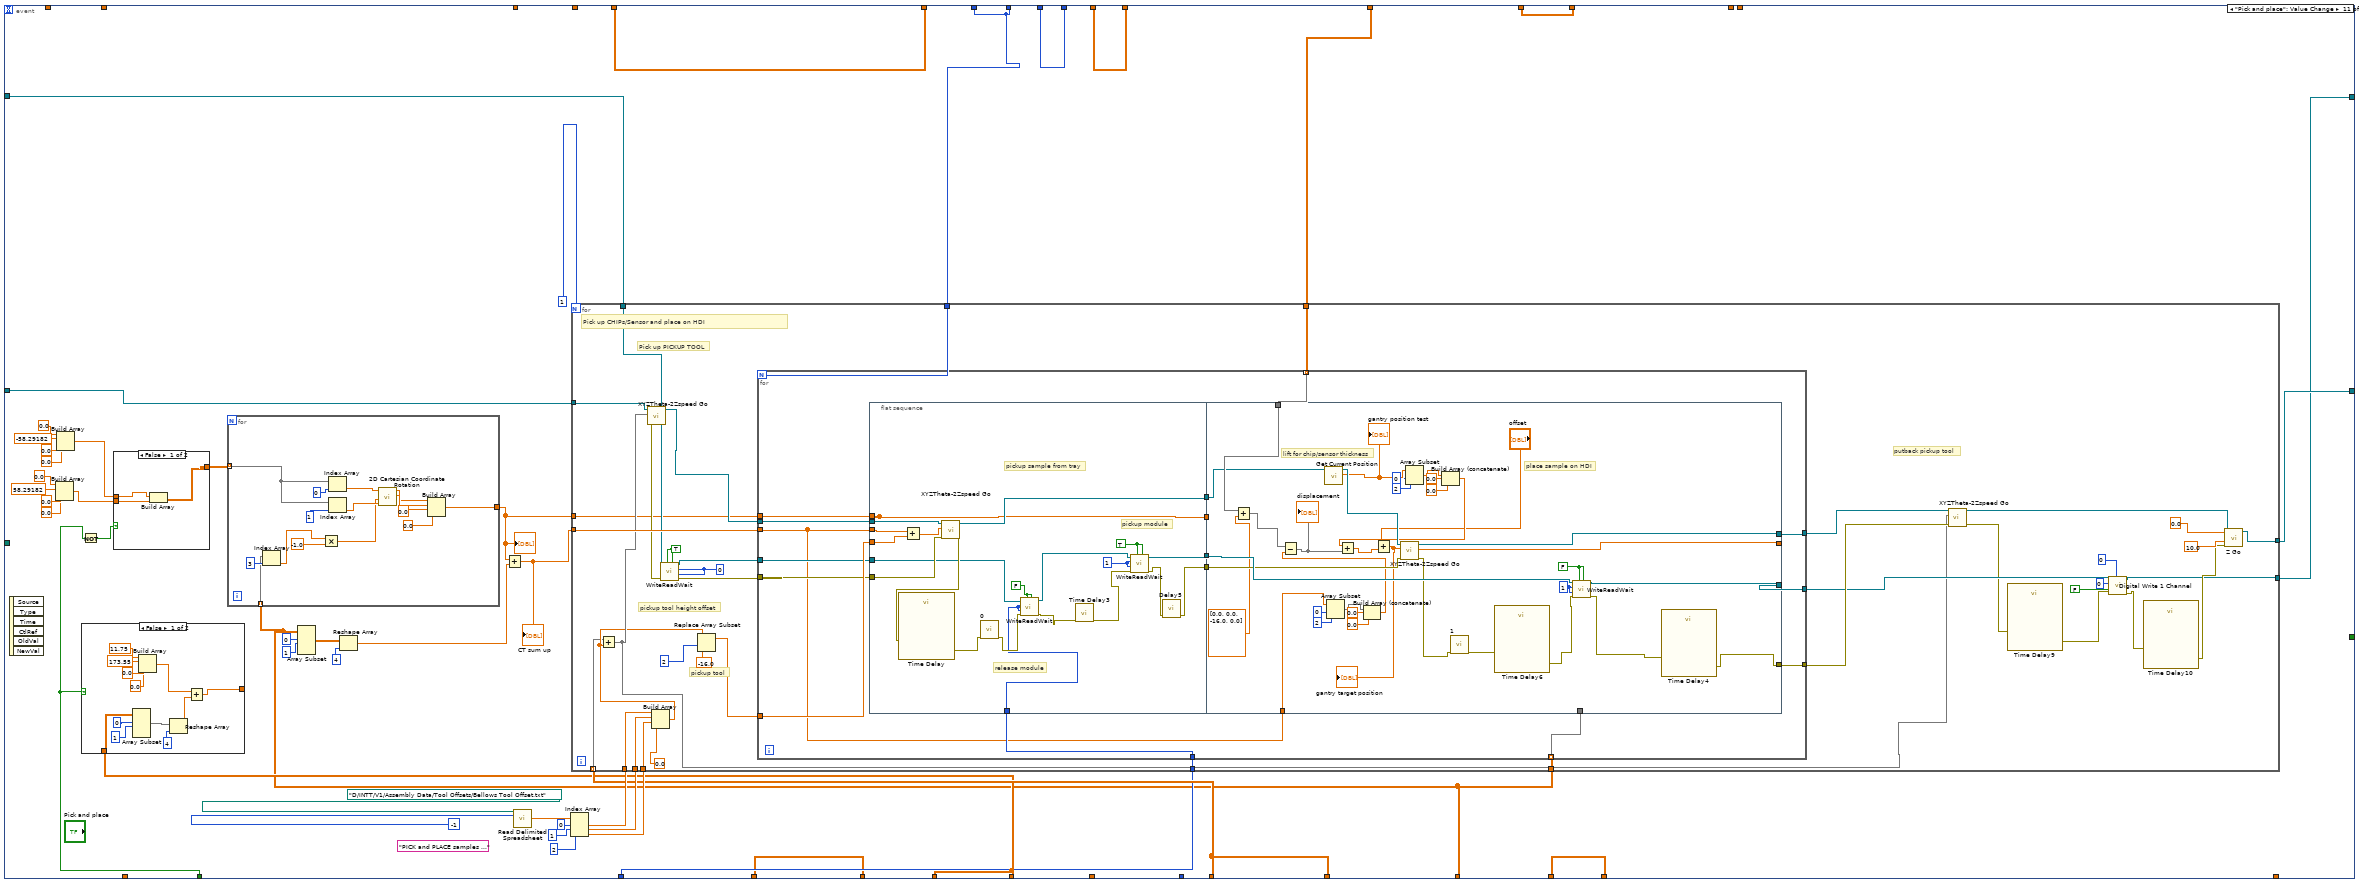
[diagram p20: hidden frame]
diagram:
  w3 = refnum<class "NI-DAQ.lvclass"> refnum  # NI-DAQ.lvclass
  n1 = call "Obtain Control Cluster.vi"("I/O"=FALSE) -> ("Control Out"=w7:T2)  [unwired: 10 in]
  n2 = Unbundle By Name(w7) -> ("Copy of Motion.lvclass"=w5:refnum<class "Motion.lvclass">)
  n3 = call-dynamic "Connect.vi"("NI-DAQ in"=w3) -> ("NI-DAQ out"=w2:refnum<class "NI-DAQ.lvclass">)  [unwired: 9 in, 1 out]
  n4 = while {
    shift-right: [w39] -> w4
    shift-left: w5 -> [w46]
    shift-right: [w19] -> w1
    shift-left: w2 -> [w23]
    i -> [w38]
    stop <- w45 stop-if-true
    # "pick&place module"
    # "default module position on stave"
    # "Pickup tool position"
    # "glue deposit module"
    # "Measured HDI geometry"
    # "module position on tray"
    # "Measured stave top-left"
    # "module on stave"
    n5 = feedback #1() -> (w43:dbl[][])  [unwired: 1 in]
    n6 = feedback #2() -> (w44:dbl[][])  [unwired: 1 in]
    n7 = feedback #3() -> (w20:dbl[][])  [unwired: 1 in]
    n8 = feedback #4() -> (w9:i32)  [unwired: 1 in]
    n9 = feedback #5() -> (w37:i32)  [unwired: 1 in]
    n10 = feedback #6() -> (w32:dbl[][])  [unwired: 1 in]
    n11 = feedback #7() -> (w40:dbl[][])  [unwired: 1 in]
    n12 = call-poly <vilib>:"Read Delimited Spreadsheet.vi"("file path (dialog if empty)"=path "D:/INTT/V1/Assembly Data/ladder assembly/2line_switch.txt" ("file path (dialog if empty) 3"), "format (%.3f)"="%.10f") -> ("all rows"=w11:dbl[][])  [unwired: 8 in, 5 out]
    "file indicator" <- w11
    n13 = feedback #8() -> (w27:dbl[][])  [unwired: 1 in]
    n14 = feedback #9() -> (w8:dbl[][])  [unwired: 1 in]
    "HDI center positions" <- w8
    n15 = event shown="[0] \"Inititalize\": Value Change" {
      selector: _ -> [_ _ _ _ _ _ _ _ _ _ _ _ _ _ _]
      dyn-events: _ -> [_ _ _ _ _ _ _ _ _ _ _ _ _ _ _]
      timeout: 500 -> [_ _ _ _ _ _ _ _ _ _ _ _ _ _ _]
      tunnel: w46 -> [w81 w121 w186 w217 w314 w413 w550 w598 w672 w830 w895 w1058 w1077 w1080 w1102]
      tunnel: [_ _ "Stop" _ _ _ _ _ _ _ _ _ _ _ _] -> w45
      tunnel: [w49 w115 w181 w188 w285 w416 w555 w593 w634 w796 w876 w1064 w1073 w1088 w1101] -> w24
      tunnel: w44 -> [_ w115 w181 _ _ _ w555 w593 w634 w796 w876 w1064 w1073 w1088 w1101]
      tunnel: [w59 w113 w180 w213 w310 w428 w559 w592 w658 w833 w878 w1061 w1072 w1082 w1099] -> w25
      tunnel: w43 -> [_ _ w180 w213 w310 w428 w559 w592 w658 w833 w878 w1061 w1072 w1082 w1099]
      tunnel: w37 -> [_ w108 w183 w218 w315 w431 w554 w589 w661 w835 w872 w1063 w1074 w1086 w1093]
      tunnel: [w64 w112 w178 w220 w317 w433 w556 w591 w660 w831 w863 w1059 w1070 w1084 w1096] -> w42
      tunnel: w8 -> [w64 _ w178 w220 w317 w433 w556 w591 w660 w831 w863 w1059 w1070 w1084 w1096]
      tunnel: [w79 w116 w179 w225 w322 w438 w557 w597 w659 w832 w884 w1060 w1071 w1083 w1097] -> w41
      tunnel: w40 -> [_ w116 w179 w225 w322 w438 w557 _ w659 w832 w884 w1060 w1071 w1083 w1097]
      tunnel: [w81 w120 w184 w214 w311 w429 w548 w596 w662 w822 w885 w1056 w1076 w1080 w1102] -> w39
      tunnel: ["deposit glue module" w108 w183 w218 w315 w431 w554 w589 w661 w835 w872 w1063 w1074 w1086 w1093] -> w36
      tunnel: "Default HDI alignment \nmark position" -> [w62 w119 _ _ _ _ _ _ _ _ _ _ _ _ _]
      tunnel: "Default HDI size" -> [w61 w118 _ _ _ _ _ _ _ _ _ _ _ _ _]
      tunnel: [w68 w117 w182 w219 w316 w432 w553 w594 w657 w834 w883 w1062 w1075 w1087 w1100] -> w33
      tunnel: w32 -> [_ w117 w182 w219 w316 w432 w553 w594 w657 w834 w883 w1062 w1075 w1087 w1100]
      tunnel: "Default Pickup Tool Position" -> [w79 _ _ _ _ _ _ w595 _ _ _ _ _ _ _]
      tunnel: "Uppler / Lower Stave" -> [w65 _ _ w198 w295 w383 _ _ w642 _ w852 _ _ _ _]
      tunnel: "Default Stave upper left mark" -> [w50 _ _ w216 w313 w415 _ _ _ _ _ _ _ _ _]
      tunnel: "Default Stave dimension" -> [w58 _ _ w215 w312 w430 _ _ _ _ _ _ _ _ _]
      tunnel: [w47 w114 w176 w197 w294 w397 w552 w590 w656 w813 w874 w1054 w1067 w1085 w1095] -> w26
      tunnel: w27 -> [w47 w114 w176 _ _ _ w552 w590 w656 w813 w874 w1054 w1067 w1085 w1095]
      tunnel: w23 -> [w57 w110 w174 w196 w293 w424 w547 w587 w651 w811 w881 w1053 w1066 w1092 w1105]
      tunnel: [w57 w110 w174 w196 w293 w424 w545 w587 w651 w811 w880 w1053 w1066 w1079 w1103] -> w19
      tunnel: "HDI vacuum channel" -> [_ _ _ _ _ _ _ _ _ _ w879 _ _ w1089 w1104]
      tunnel: [w60 w111 w175 w212 w309 w427 w558 w588 w652 w812 w877 w1055 w1068 w1081 w1098] -> w21
      tunnel: w20 -> [_ _ w175 w212 w309 w427 w558 w588 w652 w812 w877 w1055 w1068 w1081 w1098]
      tunnel: "Needle Height Compenstation\n(glue gap)" -> [_ _ _ _ _ _ _ _ w644 w804 _ _ _ _ _]
      tunnel: "Uttimus presssure" -> [_ _ _ _ _ _ _ _ w643 _ _ _ _ _ _]
      tunnel: "?" -> [_ _ _ _ _ w414 _ _ _ _ _ _ _ _ _]
      tunnel: [_ _ _ _ _ w412 _ _ _ _ _ _ _ _ _] -> _
      tunnel: "MPT offset" -> [_ _ _ _ _ w398 _ _ _ _ _ _ _ _ _]
      tunnel: w11 -> [_ _ _ _ _ _ _ _ _ _ w875 _ _ _ _]
      tunnel: [1 ("pick &place module") w109 w173 w187 w284 w394 w551 w586 w633 w794 w873 w1052 w1065 w1078 w1094] -> w10
      tunnel: w9 -> [_ w109 w173 w187 w284 w394 w551 w586 w633 w794 w873 w1052 w1065 w1078 w1094]
      tunnel: w8 -> [_ _ _ _ _ _ _ _ _ _ w853 _ _ _ _]
      tunnel: [_ _ _ _ _ w381 _ _ _ _ _ _ _ _ _] -> _
      event "Inititalize": Value Change {
        (unwired) "INITIALIZING ....." ("String")
        (unwired) "ideal delta Y between \n2 fiducial marks"
        (unwired) "ideal delta X between 2 fiducial marks"
        # "center of lower module"
        # "center of upper module"
        n16 = event-data() -> ()  [unwired: 1 in, 6 out]
        n17 = Build Array(17.0 ("element"), 411.0 ("element"), 0.0 ("element"), 0.0 ("element")) -> (w69:dbl[])
        n18 = Build Array(17.0 ("element"), 60.9 ("element"), 0.0 ("element"), 0.0 ("element")) -> (w70:dbl[])
        n19 = case shown="True" w65 {
          tunnel: w70 -> [w90 w93]
          tunnel: w69 -> [w89 w92]
          tunnel: [w88 w91] -> w68
          frame False {
            n20 = Build Array(w89, w90) -> (w88:dbl[][])
          }
          frame True {
            n21 = Build Array(w93, w92) -> (w91:dbl[][])
          }
        }
        "default module position on stave" <- w68
        n22 = Build Array(24.3 ("y"), 231.4 ("y"), 0.0 ("element"), -0.05 ("element")) -> ()  [unwired: 1 out]
        n23 = Build Array(0.0 ("element"), 238.0 ("element"), 0.0 ("element"), 0.0 ("element")) -> (w52:dbl[])
        n24 = Add(x=w50, y=w52) -> (x+y=w51:dbl[])
        n25 = Build Array(w50, w51) -> (w49:dbl[][])
        n26 = for {
          N: 2 -> [_]
          tunnel: w62 -> [w87]
          tunnel: [w87] -> w60 mode=indexing
          tunnel: w61 -> [w86]
          tunnel: [w86] -> w59 mode=indexing
        }
        n27 = Index Array(array=w58, index=3) -> (element=w66:dbl)
        n28 = for {
          tunnel: w68 -> [w101] mode=indexing
          tunnel: w66 -> [w95]
          tunnel: w50 -> [w100]
          tunnel: [w98] -> _ mode=indexing
          (unwired) 0 ("index")
          n29 = Multiply(x=w95, y=-1.0) -> (x*y=w96:dbl)
          n30 = Index Array(array=w101) -> (element=w104:dbl)  [unwired: 1 in]
          n31 = Index Array(array=w101, index=1) -> (element=w103:dbl)
          n32 = call-poly <vilib>:"2D Cartesian Coordinate Rotation.vi"("theta"=w96, "y"=w103, "x"=w104) -> ("y out"=w106:dbl, "x out"=w105:dbl)  [unwired: 6 in, 1 out]
          n33 = Build Array(w105, w106, 0.0 ("element"), 0.0 ("element")) -> (w99:dbl[])
          n34 = Add(x=w99, y=w100) -> (x+y=w98:dbl[])
        }
      }
      event "Measure HDI": Value Change {
        (unwired) "HDI alignment in progress ..." ("String")
        n35 = event-data() -> ()  [unwired: 1 in, 6 out]
        n36 = for {
          N: w109 -> [_]
          tunnel: w118 -> [w135]
          shift-right: [w132] -> w120
          shift-left: w121 -> [w133]
          tunnel: w119 -> [w134]
          tunnel: [w169] -> w111 mode=indexing
          tunnel: [w168] -> w113 mode=indexing
          tunnel: [w122] -> w112 mode=indexing
          (unwired) "ideal delta Y between \n2 fiducial marks"
          (unwired) "ideal delta X between 2 fiducial marks"
          # "1"
          # "3"
          n37 = call "Joystick and Camera SHIH VPC- external Connection.vi"("Motion in"=w133, "XYZTheta"=w134, "Measurement Point"="Measure Top-Left of HDI") -> ("Motion out"=w148:refnum<class "Motion.lvclass">, "Sum"=w125:dbl[])  [unwired: 4 in, 2 out]
          n38 = Add(x=w135, y=w125) -> (x+y=w152:dbl[])
          n39 = Index Array(array=w125, index=0) -> (element=w139:dbl)
          n40 = Array Subset(array=w152, index=0, length=2) -> (w151:dbl[])
          n41 = Replace Array Subset(array=w151, new element=w139, index=0) -> (w149:dbl[])
          n42 = call-dynamic "XY Go.vi"("Speed"=100.0, "XY"=w149, "Motion in"=w148) -> ("Motion out"=w156:refnum<class "Motion.lvclass">)  [unwired: 7 in, 1 out]
          n43 = Build Array(24.3 ("y"), 231.4 ("y"), 0.0 ("element"), -0.05 ("element")) -> ()  [unwired: 1 out]
          n44 = call "Joystick and Camera SHIH VPC- external Connection.vi"("Motion in"=w156, "Measurement Point"="Measure Bottom-Left of HDI", "Inital GO"=FALSE) -> ("Motion out"=w147:refnum<class "Motion.lvclass">, "Sum"=w138:dbl[])  [unwired: 4 in, 2 out]
          n45 = Array Subset(array=w152, index=0, length=2) -> (w162:dbl[])
          n46 = Subtract(x=w138, y=w125) -> (x-y=w146:dbl[])
          n47 = call-dynamic "XY Go.vi"("Speed"=100.0, "XY"=w162, "Motion in"=w147) -> ("Motion out"=w166:refnum<class "Motion.lvclass">)  [unwired: 7 in, 1 out]
          n48 = call "XY_to_Rotation_RPHI.vi"("X-Y"=w146) -> ("r-phi"=w142:dbl[])
          n49 = call "Joystick and Camera SHIH VPC- external Connection.vi"("Motion in"=w166, "Measurement Point"="Measure Bottom-Righ of HDI", "Inital GO"=FALSE) -> ("Motion out"=w132:refnum<class "Motion.lvclass">, "Sum"=w129:dbl[])  [unwired: 4 in, 2 out]
          n50 = Subtract(x=w129, y=w125) -> (x-y=w130:dbl[])
          n51 = Index Array(array=w142, index=1) -> (element=w136:dbl)
          n52 = Multiply(x=w136, y=-1.0) -> (x*y=w127:dbl)
          n53 = Replace Array Subset(array=w130, new element=w127, index=3) -> (w168:dbl[])
          n54 = Replace Array Subset(array=w125, new element=w127, index=3) -> (w169:dbl[])
          n55 = Add(x=w129, y=w125) -> (x+y=w171:dbl[])
          n56 = Divide(x=w171, y=2.0) -> (x/y=w126:dbl[])
          n57 = Replace Array Subset(array=w126, new element=w127, index=3) -> (w123:dbl[])
          n58 = Subtract(x=w123, y=dbl[] [0.4, 0.4, 0.0, 0.0]) -> (x-y=w122:dbl[])
        }
      }
      event "Stop": Value Change {
        n59 = event-data() -> ()  [unwired: 1 in, 6 out]
        n60 = call "XYZTheta Go.vi"("XYZTheta In"=dbl[] [625.0, 625.0, 0.0, 0.01], "Motion in"=w186) -> ("Motion out"=w184:refnum<class "Motion.lvclass">)  [unwired: 7 in, 2 out]
      }
      event "Align Stave": Value Change {
        # "center of lower module"
        # "center of upper module"
        # "Default stave dimension\namong mounting holes"
        # "Measure 2 module positions on stave"
        n61 = event-data() -> ()  [unwired: 1 in, 6 out]
        n62 = Build Array(34.0 ("element"), 470.0 ("element"), 0.0 ("element"), 0.0 ("element")) -> ()  [unwired: 1 out]
        n63 = for {
          N: 1 -> [_]
          tunnel: w215 -> [w232]
          shift-right: [w242] -> w214
          shift-left: w217 -> [w243]
          tunnel: w216 -> [w244]
          tunnel: [w237] -> w190
          tunnel: [w235] -> w200
          (unwired) "ideal delta Y between \n2 fiducial marks"
          (unwired) "ideal delta X between 2 fiducial marks"
          n64 = call "Joystick and Camera SHIH VPC- external Connection.vi"("Motion in"=w243, "XYZTheta"=w244, "Measurement Point"="Measure Top-Left of stave") -> ("Motion out"=w226:refnum<class "Motion.lvclass">, "Sum"=w228:dbl[])  [unwired: 4 in, 2 out]
          n65 = Replace Array Subset(array=w232, new element=0.0 ("new element/subarray"), index=0) -> (w229:dbl[])
          n66 = Add(x=w228, y=w229) -> (x+y=w227:dbl[])
          n67 = call "Joystick and Camera SHIH VPC- external Connection.vi"("Motion in"=w226, "XYZTheta"=w227, "Measurement Point"="Measure Bottom-Left of stave", "Inital GO"=TRUE) -> ("Motion out"=w234:refnum<class "Motion.lvclass">, "Sum"=w247:dbl[])  [unwired: 3 in, 2 out]
          n68 = Build Array(24.3 ("y"), 231.4 ("y"), 0.0 ("element"), -0.05 ("element")) -> ()  [unwired: 1 out]
          n69 = Add(x=w232, y=w228) -> (x+y=w233:dbl[])
          n70 = Subtract(x=w247, y=w228) -> (x-y=w253:dbl[])
          n71 = call "XY_to_Rotation_RPHI.vi"("X-Y"=w253) -> ("r-phi"=w249:dbl[])
          n72 = Index Array(array=w249, index=1) -> (element=w245:dbl)
          n73 = call "Joystick and Camera SHIH VPC- external Connection.vi"("Motion in"=w234, "XYZTheta"=w233, "Measurement Point"="Measure Bottom-Righ of stave", "Inital GO"=TRUE) -> ("Motion out"=w242:refnum<class "Motion.lvclass">, "Sum"=w239:dbl[])  [unwired: 3 in, 2 out]
          n74 = Subtract(x=w239, y=w228) -> (x-y=w240:dbl[])
          n75 = Multiply(x=w245, y=-1.0) -> (x*y=w235:dbl)
          n76 = Replace Array Subset(array=w240, new element=w235, index=3) -> (→"measured stave size":dbl[])
          n77 = Replace Array Subset(array=w228, new element=w235, index=3) -> (w237:dbl[])
          n78 = Add(x=w239, y=w228) -> (x+y=w261:dbl[])
          n79 = Divide(x=w261, y=2.0) -> (x/y=→"Center of module on stave":dbl[])
        }
        n80 = Build Array(0.0 ("element"), 238.0 ("element"), 0.0 ("element"), 0.0 ("element")) -> (w191:dbl[])
        n81 = Add(x=w190, y=w191) -> (x+y=w189:dbl[])
        n82 = Build Array(w190, w189) -> (w188:dbl[][])
        n83 = Build Array(17.0 ("element"), 411.0 ("element"), 0.0 ("element"), 0.0 ("element")) -> (w202:dbl[])
        n84 = Build Array(17.0 ("element"), 60.9 ("element"), 0.0 ("element"), 0.0 ("element")) -> (w203:dbl[])
        n85 = case shown="True" w198 {
          tunnel: w203 -> [w280 w283]
          tunnel: w202 -> [w279 w282]
          tunnel: [w278 w281] -> w201
          frame False {
            n86 = Build Array(w279, w280) -> (w278:dbl[][])
          }
          frame True {
            n87 = Build Array(w283, w282) -> (w281:dbl[][])
          }
        }
        n88 = for {
          tunnel: w201 -> [w271] mode=indexing
          tunnel: w200 -> [w266]
          tunnel: w190 -> [w270]
          tunnel: [w268] -> w197 mode=indexing
          n89 = Multiply(x=w266, y=-1.0) -> (x*y=w265:dbl)
          n90 = Index Array(array=w271, index=0) -> (element=w274:dbl)
          n91 = Index Array(array=w271, index=1) -> (element=w273:dbl)
          n92 = call-poly <vilib>:"2D Cartesian Coordinate Rotation.vi"("theta"=w265, "y"=w273, "x"=w274) -> ("y out"=w276:dbl, "x out"=w275:dbl)  [unwired: 6 in, 1 out]
          n93 = Build Array(w275, w276, 0.0 ("element"), 0.0 ("element")) -> (w269:dbl[])
          n94 = Add(x=w269, y=w270) -> (x+y=w268:dbl[])
        }
      }
      event "Align Stave in detail": Value Change {
        # "center of lower module"
        # "center of upper module"
        # "Default stave dimension\namong mounting holes"
        # "Measure 2 module positions on stave"
        n95 = event-data() -> ()  [unwired: 1 in, 6 out]
        n96 = Build Array(34.0 ("element"), 470.0 ("element"), 0.0 ("element"), 0.0 ("element")) -> ()  [unwired: 1 out]
        n97 = for {
          N: 1 -> [_]
          tunnel: w312 -> [w329]
          shift-right: [w339] -> w311
          shift-left: w314 -> [w340]
          tunnel: w313 -> [w341]
          tunnel: [w334] -> w287
          tunnel: [w332] -> w297
          (unwired) "ideal delta Y between \n2 fiducial marks"
          (unwired) "ideal delta X between 2 fiducial marks"
          n98 = call "Joystick and Camera SHIH V5- external Connection.vi"("Motion in"=w340, "XYZTheta"=w341, "Measurement Point"="Measure Top-Left of stave") -> ("final out"=w325:dbl[], "Motion out"=w323:refnum<class "Motion.lvclass">)  [unwired: 5 in, 1 out]
          n99 = Replace Array Subset(array=w329, new element=0.0 ("new element/subarray"), index=0) -> (w326:dbl[])
          n100 = Add(x=w325, y=w326) -> (x+y=w324:dbl[])
          n101 = call "Joystick and Camera SHIH V5- external Connection.vi"("Motion in"=w323, "XYZTheta"=w324, "Measurement Point"="Measure Bottom-Left of stave", "Inital GO"=TRUE) -> ("final out"=w344:dbl[], "Motion out"=w331:refnum<class "Motion.lvclass">)  [unwired: 4 in, 1 out]
          n102 = Build Array(24.3 ("y"), 231.4 ("y"), 0.0 ("element"), -0.05 ("element")) -> ()  [unwired: 1 out]
          n103 = Add(x=w329, y=w325) -> (x+y=w330:dbl[])
          n104 = Subtract(x=w344, y=w325) -> (x-y=w350:dbl[])
          n105 = call "XY_to_Rotation_RPHI.vi"("X-Y"=w350) -> ("r-phi"=w346:dbl[])
          n106 = Index Array(array=w346, index=1) -> (element=w342:dbl)
          n107 = call "Joystick and Camera SHIH V5- external Connection.vi"("Motion in"=w331, "XYZTheta"=w330, "Measurement Point"="Measure Bottom-Righ of stave", "Inital GO"=TRUE) -> ("final out"=w336:dbl[], "Motion out"=w339:refnum<class "Motion.lvclass">)  [unwired: 4 in, 1 out]
          n108 = Subtract(x=w336, y=w325) -> (x-y=w337:dbl[])
          n109 = Multiply(x=w342, y=-1.0) -> (x*y=w332:dbl)
          n110 = Replace Array Subset(array=w337, new element=w332, index=3) -> (→"FROM Detail !! measured stave size":dbl[])
          n111 = Replace Array Subset(array=w325, new element=w332, index=3) -> (w334:dbl[])
          n112 = Add(x=w336, y=w325) -> (x+y=w358:dbl[])
          n113 = Divide(x=w358, y=2.0) -> (x/y=→"FROM Detail !!! Center of module on stave":dbl[])
        }
        n114 = Build Array(0.0 ("element"), 238.0 ("element"), 0.0 ("element"), 0.0 ("element")) -> (w288:dbl[])
        n115 = Add(x=w287, y=w288) -> (x+y=w286:dbl[])
        n116 = Build Array(w287, w286) -> (w285:dbl[][])
        n117 = Build Array(17.0 ("element"), 411.0 ("element"), 0.0 ("element"), 0.0 ("element")) -> (w299:dbl[])
        n118 = Build Array(17.0 ("element"), 60.9 ("element"), 0.0 ("element"), 0.0 ("element")) -> (w300:dbl[])
        n119 = case shown="True" w295 {
          tunnel: w300 -> [w377 w380]
          tunnel: w299 -> [w376 w379]
          tunnel: [w375 w378] -> w298
          frame False {
            n120 = Build Array(w376, w377) -> (w375:dbl[][])
          }
          frame True {
            n121 = Build Array(w380, w379) -> (w378:dbl[][])
          }
        }
        n122 = for {
          tunnel: w298 -> [w368] mode=indexing
          tunnel: w297 -> [w363]
          tunnel: w287 -> [w367]
          tunnel: [w365] -> w294 mode=indexing
          n123 = Multiply(x=w363, y=-1.0) -> (x*y=w362:dbl)
          n124 = Index Array(array=w368, index=0) -> (element=w371:dbl)
          n125 = Index Array(array=w368, index=1) -> (element=w370:dbl)
          n126 = call-poly <vilib>:"2D Cartesian Coordinate Rotation.vi"("theta"=w362, "y"=w370, "x"=w371) -> ("y out"=w373:dbl, "x out"=w372:dbl)  [unwired: 6 in, 1 out]
          n127 = Build Array(w372, w373, 0.0 ("element"), 0.0 ("element")) -> (w366:dbl[])
          n128 = Add(x=w366, y=w367) -> (x+y=w365:dbl[])
        }
      }
      event "Bless from OGP": Value Change {
        # "center of upper module"
        # "center of lower module"
        # "center of upper module"
        # "NL line with correct rotation"
        # "Default stave dimension\namong mounting holes"
        # "Measure 2 module positions on stave"
        n129 = event-data() -> ()  [unwired: 1 in, 6 out]
        n130 = Build Array(34.0 ("element"), 470.0 ("element"), 0.0 ("element"), 0.0 ("element")) -> ()  [unwired: 1 out]
        n131 = for {
          N: 1 -> [_]
          tunnel: w430 -> [_]
          shift-right: [w490] -> w429
          shift-left: w413 -> [w503]
          tunnel: w415 -> [_]
          tunnel: [w482] -> w418
          tunnel: [w485] -> w426
          tunnel: w414 -> [w492]
          tunnel: [w468] -> w401
          (unwired) FALSE ("Inital GO")
          (unwired) "ideal delta Y between \n2 fiducial marks"
          (unwired) "ideal delta X between 2 fiducial marks"
          # "after NL"
          # "after SL"
          # "NL line"
          # "rotation"
          n132 = call "Joystick and Camera SHIH VPC- external Connection.vi"("Motion in"=w503, "XYZTheta"=dbl[] [576.333, 663.131, 70.7812, 0.010000094994154989] ("N chip"), "Measurement Point"="north chip", "Inital GO"=TRUE) -> ("Motion out"=w500:refnum<class "Motion.lvclass">, "Sum"=w480:dbl[])  [unwired: 3 in, 2 out]
          "N chip" <- w480
          n133 = call "Joystick and Camera SHIH VPC- external Connection.vi"("Motion in"=w500, "XYZTheta"=dbl[] [578.791, 1154.64, 70.5935, 0.010000670236950445] ("S chip"), "Measurement Point"="south chip", "Inital GO"=TRUE) -> ("Motion out"=w499:refnum<class "Motion.lvclass">, "Sum"=w481:dbl[])  [unwired: 3 in, 2 out]
          "S chip" <- w481
          n134 = Subtract(x=w481, y=w480) -> (x-y=w479:dbl[])
          n135 = Index Array(array=w479, index #1=0 ("index"), index #2=1 ("index")) -> (element #1=w476:dbl, element #2=w475:dbl)
          n136 = Square(x=w476) -> (x^2=w473:dbl)
          n137 = Square(x=w475) -> (x^2=w474:dbl)
          n138 = Add(x=w473, y=w474) -> (x+y=w472:dbl)
          n139 = call "Joystick and Camera SHIH VPC- external Connection.vi"("Motion in"=w499, "Measurement Point"="height of stave", "Inital GO"=FALSE) -> ("Motion out"=w490:refnum<class "Motion.lvclass">, "Sum"=w491:dbl[])  [unwired: 4 in, 2 out]
          n140 = call "O to G peek.vi"("height"=w491, "south chip"=w481, "north chip"=w480, "Input file"=w492) -> ("OGP length"=→"chip distance by OGP":dbl, "output BR"=w494:dbl[], "output BL"=w493:dbl[], "output TL"=w487:dbl[])  [unwired: 4 in]
          "after NL" <- w487
          "after SR" <- w494
          "after SL" <- w493
          n141 = Square Root(x=w472) -> (sqrt(x)=→"chip distance by gantry":dbl)
          n142 = Subtract(x=w494, y=w487) -> (x-y=w505:dbl[])
          n143 = Build Array(24.3 ("y"), 231.4 ("y"), 0.0 ("element"), -0.05 ("element")) -> ()  [unwired: 1 out]
          n144 = Subtract(x=w493, y=w487) -> (x-y=w511:dbl[])
          n145 = call "XY_to_Rotation_RPHI.vi"("X-Y"=w511) -> ("r-phi"=w510:dbl[])
          n146 = Index Array(array=w510, index=1) -> (element=w507:dbl)
          n147 = Multiply(x=w507, y=-1.0) -> (x*y=w485:dbl)
          n148 = Replace Array Subset(array=w505, new element=w485, index=3) -> (→"bless from OGP !! measured stave size":dbl[])
          n149 = Replace Array Subset(array=w487, new element=w485, index=3) -> (w483:dbl[])
          n150 = Add(x=w494, y=w487) -> (x+y=w517:dbl[])
          n151 = Divide(x=w517, y=2.0) -> (x/y=w469:dbl[])
          n152 = Add(x=w483, y=dbl[] [0.0, 10.0, 0.0, 0.0]) -> (x+y=w482:dbl[])
          n153 = Replace Array Subset(array=w469, new element=w485, index=3) -> (w468:dbl[])
          "bless from OGP !!! Center of  stave" <- w468
        }
        n154 = Build Array(0.0 ("element"), 238.0 ("element"), 0.0 ("element"), 0.0 ("element")) -> (w419:dbl[])
        n155 = Add(x=w418, y=w419) -> (x+y=w417:dbl[])
        n156 = Build Array(w418, w417) -> (w416:dbl[][])
        n157 = Build Array(0.0 ("element"), 174.94182 ("element"), 0.0 ("element"), 0.0 ("element")) -> (w402:dbl[])
        n158 = Build Array(0.0 ("element"), -174.94182 ("element"), 0.0 ("element"), 0.0 ("element")) -> (w403:dbl[])
        n159 = Build Array(0.0 ("element"), 116.65 ("element"), 0.0 ("element"), 0.0 ("element")) -> (w384:dbl[])
        n160 = Build Array(0.0 ("element"), -116.65 ("element"), 0.0 ("element"), 0.0 ("element")) -> (w385:dbl[])
        n161 = case shown="False" w383 {
          tunnel: w403 -> [w464 w467]
          tunnel: w402 -> [w463 w466]
          tunnel: [w462 w465] -> w400
          frame False {
            n162 = Build Array(w463, w464) -> (w462:dbl[][])
          }
          frame True {
            n163 = Build Array(w467, w466) -> (w465:dbl[][])
          }
        }
        n164 = case shown="True" w383 {
          tunnel: w385 -> [w441 w444]
          tunnel: w384 -> [w440 w443]
          tunnel: [w439 w442] -> w382
          frame False {
            n165 = Build Array(w440, w441) -> (w439:dbl[][])
          }
          frame True {
            n166 = Build Array(w444, w443) -> (w442:dbl[][])
          }
        }
        n167 = for {
          tunnel: w400 -> [w538] mode=indexing
          tunnel: w426 -> [w535]
          tunnel: [w537] -> w412 mode=indexing
          tunnel: w401 -> [w520]
          tunnel: [w532] -> w399 mode=indexing
          tunnel: w382 -> [w523] mode=indexing
          tunnel: [w519] -> w381 mode=indexing
          n168 = Multiply(x=w535, y=-1.0) -> (x*y=w522:dbl)
          n169 = Index Array(array=w538, index=0) -> (element=w541:dbl)
          n170 = Index Array(array=w538, index=1) -> (element=w540:dbl)
          n171 = Index Array(array=w523, index=0) -> (element=w528:dbl)
          n172 = Index Array(array=w523, index=1) -> (element=w527:dbl)
          n173 = call-poly <vilib>:"2D Cartesian Coordinate Rotation.vi"("theta"=w522, "y"=w540, "x"=w541) -> ("y out"=w543:dbl, "x out"=w542:dbl)  [unwired: 6 in, 1 out]
          n174 = call-poly <vilib>:"2D Cartesian Coordinate Rotation.vi"("theta"=w522, "y"=w527, "x"=w528) -> ("y out"=w530:dbl, "x out"=w529:dbl)  [unwired: 6 in, 1 out]
          n175 = Build Array(w542, w543, 0.0 ("element"), 0.0 ("element")) -> (w532:dbl[])
          n176 = Build Array(w529, w530, 0.0 ("element"), 0.0 ("element")) -> (w521:dbl[])
          n177 = Add(x=w521, y=w520) -> (x+y=w519:dbl[])
          n178 = Add(x=w532, y=w520) -> (x+y=w537:dbl[])
        }
        "CT HPoS" <- w399
        "HDI center positions" <- w381
        n179 = Add(x=w412, y=w398) -> (x+y=w397:dbl[][])
        n180 = call-poly <vilib>:"Write Delimited Spreadsheet.vi"("file path (dialog if empty)"=path "D:/INTT/V1/Assembly Data/ladder assembly/2line_switch.txt", "format (%.3f)"="%.10f", "2D data"=w397) -> ()  [unwired: 11 in, 2 out]
        n181 = disable-structure shown="Disabled" {
          disable-tunnel: w383 -> [w445 _]
          frame Disabled {
            # "center of lower module"
            # "center of upper module"
            n182 = Build Array(17.0 ("element"), 60.9 ("element"), 0.0 ("element"), 0.0 ("element")) -> (w447:dbl[])
            n183 = Build Array(17.0 ("element"), 411.0 ("element"), 0.0 ("element"), 0.0 ("element")) -> (w446:dbl[])
            n184 = case shown="True" w445 {
              tunnel: w447 -> [w458 w461]
              tunnel: w446 -> [w457 w460]
              tunnel: [w456 w459] -> _
              frame False {
                n185 = Build Array(w457, w458) -> (w456:dbl[][])
              }
              frame True {
                n186 = Build Array(w461, w460) -> (w459:dbl[][])
              }
            }
          }
          frame Enabled {
          }
        }
      }
      event "txt switch": Value Change {
        n187 = event-data() -> ()  [unwired: 1 in, 6 out]
        n188 = flat-sequence {
          tunnel: [w566] -> w560
          tunnel: w550 -> [w562]
          tunnel: [w562] -> w549
          tunnel: w547 -> [w561]
          tunnel: [w561] -> w546
          tunnel: w560 -> [w584]
          tunnel: [w582] -> w548
          tunnel: w549 -> [w582]
          tunnel: [w581] -> w545
          tunnel: w546 -> [w581]
          frame #0 {
            n189 = call-poly <vilib>:"Read Delimited Spreadsheet.vi"("file path (dialog if empty)"=path "D:/INTT/V1/Assembly Data/ladder assembly/2line_switch.txt" ("file path (dialog if empty) 3"), "format (%.3f)"="%.10f") -> ("all rows"=w567:dbl[][])  [unwired: 8 in, 5 out]
            n190 = Array Subset(array=w567, index (row)=0 ("index"), length (row)=1 ("length"), index (col)=0 ("index"), length (col)=4 ("length")) -> (w577:dbl[][])
            n191 = Reshape Array(w577, 4 ("dimension size")) -> (w564:dbl[])
            n192 = Array Subset(array=w567, index (row)=1 ("index"), length (row)=1 ("length"), index (col)=0 ("index"), length (col)=4 ("length")) -> (w571:dbl[][])
            n193 = Reshape Array(w571, 4 ("dimension size")) -> (w565:dbl[])
            n194 = Build Array(w565, w564) -> (w566:dbl[][])
          }
          frame #1 {
            n195 = call-poly <vilib>:"Write Delimited Spreadsheet.vi"("file path (dialog if empty)"=path "D:/INTT/V1/Assembly Data/ladder assembly/2line_switch.txt" ("file path (dialog if empty) 4"), "format (%.3f)"="%.10f", "2D data"=w584) -> ()  [unwired: 11 in, 2 out]
          }
        }
      }
      event "Measure Pickup Tools": Value Change {
        (unwired) "Measuring Pickup Tools" ("String")
        n196 = event-data() -> ()  [unwired: 1 in, 6 out]
        n197 = for {
          N: w586 -> [_]
          tunnel: [w622] -> w597 mode=indexing
          tunnel: w598 -> [w626]
          tunnel: [w608] -> w596
          tunnel: w595 -> [w607] mode=indexing
          # "Default size and\norientation"
          n198 = call "Joystick and Camera SHIH VPC- external Connection.vi"("Motion in"=w626, "XYZTheta"=w607, "Measurement Point"="PickUp tool Top") -> ("Motion out"=w602:refnum<class "Motion.lvclass">, "Sum"=w625:dbl[])  [unwired: 4 in, 2 out]
          n199 = Build Array(0.0 ("element"), 29.94 ("element"), 0.0 ("element"), 0.0 ("element")) -> (w613:dbl[])
          n200 = Add(x=w625, y=w613) -> (x+y=w599:dbl[])
          n201 = Array Subset(array=w599, index=0, length=2) -> (w600:dbl[])
          n202 = call-dynamic "XY Go.vi"("Speed"=20.0, "XY"=w600, "Motion in"=w602) -> ("Motion out"=w601:refnum<class "Motion.lvclass">)  [unwired: 7 in, 1 out]
          n203 = call "Joystick and Camera SHIH VPC- external Connection.vi"("Motion in"=w601, "Measurement Point"="PickUp tool Bottom", "Inital GO"=FALSE) -> ("Motion out"=w608:refnum<class "Motion.lvclass">, "Sum"=w624:dbl[])  [unwired: 4 in, 2 out]
          n204 = Add(x=w625, y=w624) -> (x+y=w631:dbl[])
          n205 = Subtract(x=w624, y=w625) -> (x-y=w623:dbl[])
          n206 = Divide(x=w631, y=2.0) -> (x/y=w628:dbl[])
          n207 = call "XYtoRPHI.vi"("X-Y"=w623) -> ("r-phi"=w629:dbl[])
          n208 = Index Array(array=w629, index=1) -> (element=w617:dbl)
          n209 = Absolute Value(x=w617) -> (abs(x)=w620:dbl)
          n210 = Sign(1:w617) -> (0:w618:dbl)
          n211 = Subtract(x=w620, y=1.5707963267948966) -> (x-y=w619:dbl)
          n212 = Multiply(x=w618, y=w619) -> (x*y=w616:dbl)
          n213 = Replace Array Subset(array=w628, new element=w616, index=3) -> (w622:dbl[])
          "PickupTool \nCenterPosition" <- w622
        }
      }
      event "Deposit Glue": Value Change {
        # "CF height"
        # "surface z offset"
        # "two sensor, Sensor B then A"
        # "Unmount syringe"
        # "first needle park position\nneedle gap on Z value : 0.5 mm"
        # "Syringe-camera offset"
        n214 = event-data() -> ()  [unwired: 1 in, 6 out]
        n215 = call-poly <vilib>:"Read Delimited Spreadsheet.vi"("file path (dialog if empty)"=path "D:/INTT/V1/Assembly Data/Tool Offsets/Dispense Tip Offset.txt", "number of rows (all:-1)"=-1) -> ("first row"=w688:dbl[])  [unwired: 8 in, 5 out]
        n216 = Add(x=14.2 ("element"), y=w644) -> (x+y=w638:dbl)
        n217 = Index Array(array=w688, index #1=0 ("index"), index #2=1 ("index")) -> (element #1=w683:dbl, element #2=w681:dbl)
        n218 = Build Array(w683, w681, 0.0 ("element"), 0.0 ("element")) -> (w667:dbl[])
        n219 = Array Subset(array=w634, index (row)=0, length (row)=1 ("length")) -> (w647:dbl[][])  [unwired: 2 in]
        n220 = Reshape Array(w647, 4 ("dimension size")) -> (w640:dbl[])
        n221 = Index Array(array=w640, index=2) -> (element=w635:dbl)
        n222 = Add(x=w635, y=w638) -> (x+y=w637:dbl)
        n223 = Build Array(436.638, 1040.76, w637, 0.0 ("element")) -> (w636:dbl[])
        "Needle parking position" <- w636
        n224 = call "XYZTheta Go.vi"("XYZTheta In"=w636, "Motion in"=w672) -> ("error out"=w680:errorcluster, "Motion out"=w671:refnum<class "Motion.lvclass">)  [unwired: 7 in, 1 out]
        n225 = call "Display Message to User"("error in (no error)"=w680) -> ("error out"=w673:errorcluster)  [unwired: 9 in, 1 out]
        n226 = case shown="False" w642 {
          tunnel: w634 -> [w696 w705]
          tunnel: [w693 w705] -> w641
          frame False {
            n227 = Array Subset(array=w696, index (row)=1 ("index"), length (row)=1 ("length")) -> (w697:dbl[][])  [unwired: 2 in]
            n228 = Array Subset(array=w696, index (row)=0 ("index"), length (row)=1 ("length")) -> (w700:dbl[][])  [unwired: 2 in]
            n229 = Reshape Array(w700, 4 ("dimension size")) -> (w695:dbl[])
            n230 = Reshape Array(w697, 4 ("dimension size")) -> (w694:dbl[])
            n231 = Build Array(w694, w695) -> (w693:dbl[][])
          }
          frame True {
          }
        }
        n232 = call-dynamic "Z Go.vi"("error in (no error)"=w673, "Speed"=20.0, "Position"=0.0, "Motion in"=w671) -> ("error out"=w670:errorcluster, "Motion out"=w676:refnum<class "Motion.lvclass">)  [unwired: 6 in]
        n233 = call "Display Message to User2"("error in (no error)"=w670) -> ("error out"=w669:errorcluster)  [unwired: 9 in, 1 out]
        n234 = Add(x=w635, y=-2.5) -> (x+y=w677:dbl)
        n235 = call-dynamic "Z Go.vi"("error in (no error)"=w669, "Speed"=20.0, "Position"=w677, "Motion in"=w676) -> ("error out"=w646:errorcluster, "Motion out"=w668:refnum<class "Motion.lvclass">)  [unwired: 6 in]
        n236 = call-dynamic "Connect.vi"("Ultimus V in"=refnum<class "Ultimus V2.lvclass"> refnum ("Ultimus V2.lvclass")) -> ("Ultimus V out"=w666:refnum<class "Ultimus V2.lvclass">)  [unwired: 9 in, 1 out]
        n237 = for {
          N: w661 -> [_]
          tunnel: w668 -> [w734]
          tunnel: w666 -> [w721]
          tunnel: w667 -> [w735]
          tunnel: w641 -> [w736] mode=indexing
          tunnel: [w733] -> w654
          tunnel: [w732] -> w653
          tunnel: w646 -> [w728]
          tunnel: [w729] -> w645
          tunnel: w643 -> [_]
          (unwired) 100.0 ("Speed")
          n238 = Add(x=w736, y=w735) -> (x+y=w763:dbl[])
          n239 = Add(x=w763, y=dbl[] [3.3, 5.0, 0.0, 0.0]) -> (x+y=w764:dbl[])
          n240 = Index Array(array=w764, index=2) -> (element=w726:dbl)
          n241 = Array Subset(array=w764, index=0, length=2) -> (w741:dbl[])
          n242 = call-dynamic "XY Go.vi"("error in (no error)"=w728, "Speed"=100.0, "XY"=w741, "Motion in"=w734) -> ("error out"=w724:errorcluster, "Motion out"=w725:refnum<class "Motion.lvclass">)  [unwired: 6 in]
          n243 = case shown="True" "check height?" {
            tunnel: w726 -> [_ w792]
            tunnel: w725 -> [w785 w791]
            tunnel: w724 -> [w786 w790]
            tunnel: [w786 w788] -> w723
            tunnel: [w785 w787] -> w722
            frame False {
            }
            frame True {
              n244 = call-dynamic "Z Go.vi"("error in (no error)"=w790, "Speed"=5.0, "Position"=w792, "Motion in"=w791) -> ("error out"=w789:errorcluster, "Motion out"=w787:refnum<class "Motion.lvclass">)  [unwired: 6 in]
              n245 = call "Display Message to User4"("error in (no error)"=w789) -> ("error out"=w788:errorcluster)  [unwired: 9 in, 1 out]
            }
          }
          n246 = flat-sequence {
            tunnel: w721 -> [w782]
            tunnel: [w782] -> w720
            tunnel: w720 -> [w784]
            tunnel: [w784] -> w719
            tunnel: [w783] -> w718
            frame #0 {
            }
            frame #1 {
              n247 = call "air pressure setting.vi"() -> ("air pressure indecator"=w783:i32)  [unwired: 1 out]
            }
          }
          n248 = Add(x=w726, y=-2.0) -> (x+y=w740:dbl)
          n249 = call-dynamic "Z Go.vi"("error in (no error)"=w723, "Speed"=5.0, "Position"=w740, "Motion in"=w722) -> ("error out"=w738:errorcluster, "Motion out"=w739:refnum<class "Motion.lvclass">)  [unwired: 6 in]
          n250 = call "Muliti_XY_dispense.vi"("Pressure"=w718, "Path count"=4, "distances"=dbl[][] [[0.0, 224.0], [27.4, 0.0], [0.0, -224.0], [-27.4, 0.0]], "Ultimus V in"=w719, "Motion in"=w739) -> ("Ultimus V out"=w715:refnum<class "Ultimus V2.lvclass">, "Motion out"=w762:refnum<class "Motion.lvclass">)  [unwired: 5 in]
          n251 = flat-sequence {
            tunnel: w715 -> [w779]
            tunnel: [w779] -> w717
            tunnel: w717 -> [w781]
            tunnel: [w781] -> w714
            tunnel: [w780] -> w711
            frame #0 {
            }
            frame #1 {
              n252 = call "air pressure setting.vi"() -> ("air pressure indecator"=w780:i32)  [unwired: 1 out]
            }
          }
          n253 = call-dynamic "wrtCurrent Go.vi"("axis names"=string[] ["X", "Y"], "error in (no error)"=w738, "Speed"=5.0, "distances"=dbl[] [4.6, 5.0], "Motion in"=w762) -> ("error out"=w731:errorcluster, "Motion out"=w757:refnum<class "Motion.lvclass">)  [unwired: 5 in]
          n254 = call "Muliti_XY_dispense.vi"("Pressure"=w711, "Path count"=4, "distances"=dbl[][] [[0.0, 214.0], [18.2, 0.0], [0.0, -214.0], [-18.2, 0.0]], "Ultimus V in"=w714, "Motion in"=w757) -> ("Ultimus V out"=w713:refnum<class "Ultimus V2.lvclass">, "Motion out"=w750:refnum<class "Motion.lvclass">)  [unwired: 5 in]
          n255 = call-dynamic "wrtCurrent Go.vi"("axis names"=string[] ["X", "Y"], "error in (no error)"=w731, "Speed"=5.0, "distances"=dbl[] [4.6, 5.0], "Motion in"=w750) -> ("error out"=w730:errorcluster, "Motion out"=w749:refnum<class "Motion.lvclass">)  [unwired: 5 in]
          n256 = flat-sequence {
            tunnel: w713 -> [w776]
            tunnel: [w776] -> w716
            tunnel: w716 -> [w778]
            tunnel: [w778] -> w712
            tunnel: [w777] -> w707
            frame #0 {
            }
            frame #1 {
              n257 = call "air pressure setting.vi"() -> ("air pressure indecator"=w777:i32)  [unwired: 1 out]
            }
          }
          n258 = call "Muliti_XY_dispense.vi"("Pressure"=w707, "Path count"=4, "distances"=dbl[][] [[0.0, 204.0], [9.0, 0.0], [0.0, -204.0], [-9.0, 0.0]], "Ultimus V in"=w712, "Motion in"=w749) -> ("Ultimus V out"=w709:refnum<class "Ultimus V2.lvclass">, "Motion out"=w737:refnum<class "Motion.lvclass">)  [unwired: 5 in]
          n259 = flat-sequence {
            tunnel: w709 -> [w773]
            tunnel: [w773] -> w710
            tunnel: w710 -> [w775]
            tunnel: [w775] -> w708
            tunnel: [w774] -> w706
            frame #0 {
            }
            frame #1 {
              n260 = call "air pressure setting.vi"() -> ("air pressure indecator"=w774:i32)  [unwired: 1 out]
            }
          }
          n261 = call-dynamic "wrtCurrent Go.vi"("axis names"=string[] ["X", "Y"], "error in (no error)"=w730, "Speed"=5.0, "distances"=dbl[] [4.5, 5.0], "Motion in"=w737) -> ("error out"=w729:errorcluster, "Motion out"=w743:refnum<class "Motion.lvclass">)  [unwired: 5 in]
          n262 = call "Muliti_XY_dispense.vi"("Pressure"=w706, "Path count"=1, "distances"=dbl[][] [[0.0, 194.0], [7.0, 0.0], [0.0, -206.0], [-7.0, 0.0]], "Ultimus V in"=w708, "Motion in"=w743) -> ("Ultimus V out"=w732:refnum<class "Ultimus V2.lvclass">, "Motion out"=w733:refnum<class "Motion.lvclass">)  [unwired: 5 in]
        }
        n263 = call "XYZTheta Go.vi"("error in (no error)"=w645, "XYZTheta In"=dbl[] [500.0, 1000.0, 0.0, 0.1], "Motion in"=w654) -> ("error out"=w664:errorcluster, "Motion out"=w662:refnum<class "Motion.lvclass">)  [unwired: 6 in, 1 out]
        n264 = call "Display Message to User3"("error in (no error)"=w664) -> ()  [unwired: 9 in, 2 out]
        n265 = call-dynamic "Disconnect.vi"("Ultimus V in"=w653) -> ()  [unwired: 9 in, 1 out]
      }
      event "Needle Alignment": Value Change {
        (unwired) "Needle Alignment in progress ...." ("String")
        # "CF height"
        # "surface z offset"
        # "first needle park position\nneedle gap on Z value : 0.5 mm"
        # "Syringe-camera offset"
        n266 = event-data() -> ()  [unwired: 1 in, 6 out]
        n267 = Array Subset(array=w796, index (row)=0, length (row)=1 ("length")) -> (w799:dbl[][])  [unwired: 2 in]
        n268 = Reshape Array(w799, 4 ("dimension size")) -> (w798:dbl[])
        n269 = Index Array(array=w798, index=2) -> (element=w795:dbl)
        n270 = call-poly <vilib>:"Read Delimited Spreadsheet.vi"("file path (dialog if empty)"=path "D:/INTT/V1/Assembly Data/Tool Offsets/Dispense Tip Offset.txt", "number of rows (all:-1)"=-1) -> ("first row"=w846:dbl[])  [unwired: 8 in, 5 out]
        n271 = Index Array(array=w846, index #1=0 ("index"), index #2=1 ("index")) -> (element #1=w841:dbl, element #2=w840:dbl)
        n272 = Add(x=14.2 ("element"), y=w804) -> (x+y=w806:dbl)
        n273 = Add(x=w795, y=w806) -> (x+y=w805:dbl)
        n274 = Build Array(436.638, 1040.76, w805, 0.0 ("element")) -> (w803:dbl[])
        n275 = Build Array(w841, w840, 0.0 ("element"), 0.0 ("element")) -> (w815:dbl[])
        n276 = call "XYZTheta Go.vi"("XYZTheta In"=w803, "Motion in"=w830) -> ("error out"=w839:errorcluster, "XYZTheta Out"=w820:dbl[], "Motion out"=w829:refnum<class "Motion.lvclass">)  [unwired: 7 in]
        n277 = call "Display Message to User10"("error in (no error)"=w839) -> ("error out"=w836:errorcluster)  [unwired: 9 in, 1 out]
        n278 = call-dynamic "Z Go.vi"("error in (no error)"=w836, "Speed"=20.0, "Position"=0.0, "Motion in"=w829) -> ("Motion out"=w828:refnum<class "Motion.lvclass">)  [unwired: 6 in, 1 out]
        n279 = Replace Array Subset(array=w820, new element=0.0 ("new element/subarray"), index=2) -> (w817:dbl[])
        n280 = call "Joystick and Camera SHIH VPC- external Connection.vi"("Motion in"=w828, "XYZTheta"=w817, "Measurement Point"="Touch Needle on a surface") -> ("Motion out"=w826:refnum<class "Motion.lvclass">, "Gantry"=w816:dbl[])  [unwired: 4 in, 2 out]
        n281 = Subtract(x=w816, y=w815) -> (x-y=w814:dbl[])
        n282 = call "Joystick and Camera SHIH VPC- external Connection.vi"("Motion in"=w826, "XYZTheta"=w814, "Measurement Point"="Measure the touch spot with camera") -> ("Motion out"=w822:refnum<class "Motion.lvclass">, "Gantry"=w825:dbl[])  [unwired: 4 in, 2 out]
        n283 = Subtract(x=w816, y=w825) -> (x-y=w824:dbl[])
        n284 = call-poly <vilib>:"Write Delimited Spreadsheet.vi"("file path (dialog if empty)"=path "D:/INTT/V1/Assembly Data/Tool Offsets/Dispense Tip Offset.txt", "1D data"=w824, "append to file? (new file:F)"=FALSE) -> ()  [unwired: 11 in, 2 out]
      }
      event "Pick and place": Value Change {
        (unwired) "PICK and PLACE samples ..." ("String")
        n285 = event-data() -> ()  [unwired: 1 in, 6 out]
        n286 = Build Array(0.0 ("element"), 58.29182 ("element"), 0.0 ("element"), 0.0 ("element")) -> (w858:dbl[])
        n287 = Build Array(0.0 ("element"), -58.29182 ("element"), 0.0 ("element"), 0.0 ("element")) -> (w857:dbl[])
        n288 = case shown="False" w852 {
          tunnel: w877 -> [w1029 w1051]
          tunnel: [w1028 w1050] -> _
          frame False {
            n289 = Array Subset(array=w1029, index (row)=0 ("index"), length (row)=1 ("length")) -> (w1031:dbl[][])  [unwired: 2 in]
            n290 = Build Array(11.75 ("element"), 173.55 ("element"), 0.0 ("element"), 0.0 ("element")) -> (w1035:dbl[])
            n291 = Reshape Array(w1031, 4 ("dimension size")) -> (w1030:dbl[])
            n292 = Add(x=w1035, y=w1030) -> (x+y=w1028:dbl[])
          }
          frame True {
            n293 = Array Subset(array=w1051, index (row)=0 ("index"), length (row)=1 ("length")) -> (w1041:dbl[][])  [unwired: 2 in]
            n294 = Build Array(11.75 ("element"), 56.85 ("element"), 0.0 ("element"), 0.0 ("element")) -> (w1045:dbl[])
            n295 = Reshape Array(w1041, 4 ("dimension size")) -> (w1040:dbl[])
            n296 = Add(x=w1045, y=w1040) -> (x+y=w1050:dbl[])
          }
        }
        n297 = Not(x=w852) -> (.not. x?=w851:bool)
        n298 = case shown="False" w851 {
          tunnel: w858 -> [w1022 w1025]
          tunnel: w857 -> [w1023 w1026]
          tunnel: [w1024 w1027] -> w856
          frame False {
            n299 = Build Array(w1023, w1022) -> (w1024:dbl[][])
          }
          frame True {
            n300 = Build Array(w1025, w1026) -> (w1027:dbl[][])
          }
        }
        n301 = for {
          tunnel: [w901] -> w850
          tunnel: w856 -> [w900] mode=indexing
          tunnel: w853 -> [w897] mode=indexing
          n302 = Index Array(array=w897, index=3) -> (element=w898:dbl)
          n303 = Multiply(x=w898, y=-1.0) -> (x*y=w896:dbl)
          n304 = Index Array(array=w900, index=0) -> (element=w907:dbl)
          n305 = Index Array(array=w900, index=1) -> (element=w906:dbl)
          n306 = call-poly <vilib>:"2D Cartesian Coordinate Rotation.vi"("theta"=w896, "y"=w906, "x"=w907) -> ("y out"=w909:dbl, "x out"=w908:dbl)  [unwired: 6 in, 1 out]
          n307 = Build Array(w908, w909, 0.0 ("element"), 0.0 ("element")) -> (w901:dbl[])
        }
        "?" <- w850
        n308 = Array Subset(array=w853, index (row)=0 ("index"), length (row)=1 ("length")) -> (w864:dbl[][])  [unwired: 2 in]
        n309 = Reshape Array(w864, 4 ("dimension size")) -> (w855:dbl[])
        n310 = Add(x=w850, y=w855) -> (x+y=w854:dbl[])
        "CT sum up" <- w854
        n311 = call-poly <vilib>:"Read Delimited Spreadsheet.vi"("file path (dialog if empty)"=path "D:/INTT/V1/Assembly Data/Tool Offsets/Bellows Tool Offset.txt", "number of rows (all:-1)"=-1) -> ("first row"=w892:dbl[])  [unwired: 8 in, 5 out]
        n312 = Index Array(array=w892, index #1=0 ("index"), index #2=1 ("index"), index #3=2 ("index")) -> (element #1=w888:dbl, element #2=w887:dbl, element #3=w886:dbl)
        n313 = for {
          N: 1 -> [_]
          tunnel: w895 -> [w920]
          tunnel: [w941] -> w885
          tunnel: w884 -> [w913] mode=indexing
          tunnel: [w929] -> w880
          tunnel: w881 -> [w919]
          tunnel: w888 -> [w943]
          tunnel: w887 -> [w942]
          tunnel: w886 -> [w940]
          tunnel: w873 -> [w935]
          tunnel: w879 -> [w922]
          tunnel: w854 -> [w921]
          tunnel: w875 -> [w917]
          tunnel: w853 -> [w912]
          tunnel: w850 -> [w911]
          w931 = 0 ("Write")
          w934 = TRUE ("Write Value")
          # "putback pickup tool"
          # "pickup tool"
          # "pickup tool height offset"
          # "Pick up PICKUP TOOL"
          # "Pick up CHIPs/Sensor and place on HDI"
          n314 = Build Array(w943, w942, w940, 0.0 ("element")) -> (w914:dbl[])
          n315 = Add(x=w913, y=w914) -> (x+y=w915:dbl[])
          n316 = call "XYZTheta-2Zspeed Go.vi"("XYZTheta In"=w915, "Motion in"=w920) -> ("error out"=w918:errorcluster, "Motion out"=w916:refnum<class "Motion.lvclass">)  [unwired: 7 in, 1 out]
          n317 = call "WriteReadWait.vi"("Read Value"=w934, "Write Value"=w934, "error in (no error)"=w918, "Read"=w931, "Write"=w931, "I-O in"=w919) -> ("error out"=w933:errorcluster, "I-O out"=w932:refnum<class "NI-DAQ.lvclass">)  [unwired: 4 in]
          n318 = Replace Array Subset(array=w914, new element=-16.0 ("t"), index=2) -> (w938:dbl[])
          n319 = for {
            N: w935 -> [_]
            tunnel: w916 -> [w964]
            tunnel: w938 -> [w963]
            tunnel: w933 -> [w962]
            tunnel: [w961] -> w944
            tunnel: w932 -> [w960]
            tunnel: [w959] -> w930
            tunnel: [w958] -> w937
            tunnel: w922 -> [w955]
            tunnel: w921 -> [w952]
            tunnel: w917 -> [w954] mode=indexing
            tunnel: w912 -> [w953] mode=indexing
            tunnel: w911 -> [w951]
            n320 = flat-sequence {
              tunnel: [w986] -> w965
              tunnel: w964 -> [w985]
              tunnel: w963 -> [w984]
              tunnel: w962 -> [w982]
              tunnel: w960 -> [w976]
              tunnel: [w981] -> w957
              tunnel: [w968] -> w956
              tunnel: w955 -> [w967]
              tunnel: w952 -> [w979]
              tunnel: [w970] -> _
              tunnel: w951 -> [w970]
              tunnel: [w970] -> w950
              tunnel: w965 -> [w1010]
              tunnel: [w1021] -> w961
              tunnel: [w1020] -> _
              tunnel: [w1016] -> w959
              tunnel: [w990] -> w958
              tunnel: w957 -> [w1018]
              tunnel: w956 -> [w1014]
              tunnel: w954 -> [w1015]
              tunnel: w953 -> [_]
              tunnel: w952 -> [w992]
              tunnel: w950 -> [_]
              frame #0 {
                w974 = FALSE ("Write Value")
                w980 = TRUE ("Write Value")
                w966 = 1 ("Write")
                # "pickup module"
                # "release module"
                # "pickup sample from tray"
                n321 = Add(x=w979, y=w984) -> (x+y=w983:dbl[])
                n322 = call "XYZTheta-2Zspeed Go.vi"("error in (no error)"=w982, "XYZTheta In"=w983, "Motion in"=w985) -> ("error out"=w977:errorcluster, "Motion out"=w986:refnum<class "Motion.lvclass">)  [unwired: 6 in, 1 out]
                n323 = call "Time Delay"("error in (no error)"=w977) -> ("error out"=w971:errorcluster)  [unwired: 10 in]
                n324 = call "0"("error in (no error)"=w971) -> ("error out"=w972:errorcluster)  [unwired: 9 in, 1 out]
                n325 = call "WriteReadWait.vi"("Read Value"=w974, "Write Value"=w974, "error in (no error)"=w972, "Read"=w967, "Write"=w967, "I-O in"=w976) -> ("error out"=w973:errorcluster, "I-O out"=w975:refnum<class "NI-DAQ.lvclass">)  [unwired: 4 in]
                n326 = call "Time Delay3"("error in (no error)"=w973) -> ("error out"=w978:errorcluster)  [unwired: 10 in]
                n327 = call "WriteReadWait.vi"("Read Value"=w980, "Write Value"=w980, "error in (no error)"=w978, "Read"=w966, "Write"=w966, "I-O in"=w975) -> ("error out"=w969:errorcluster, "I-O out"=w981:refnum<class "NI-DAQ.lvclass">)  [unwired: 4 in]
                n328 = call "Delay5"("error in (no error)"=w969) -> ("error out"=w968:errorcluster)  [unwired: 10 in]
              }
              frame #1 {
                w1017 = 1 ("Write")
                w1019 = FALSE ("Write Value")
                # "lift for chip/sensor thickness"
                # "place sample on HDI"
                n329 = Add(x=w1015, y=dbl[] [0.0, 0.0, -16.0, 0.0]) -> (x+y=w1008:dbl[])
                n330 = call-dynamic "Get Current Position.vi"("Motion in"=w1010) -> ("XYZTheta Out"=w1006:dbl[], "Motion out"=w1009:refnum<class "Motion.lvclass">)  [unwired: 8 in, 1 out]
                "gantry position test" <- w1006
                n331 = Array Subset(array=w992, index=0, length=2) -> (w995:dbl[])
                n332 = Build Array (concatenate)(w995, 0.0 ("element"), 0.0 ("element")) -> (w994:dbl[])
                n333 = Subtract(x=w1008, y=w994) -> (x-y=w1007:dbl[])
                "displacement" <- w1007
                n334 = Array Subset(array=w1006, index=0, length=2) -> (w1001:dbl[])
                n335 = Build Array (concatenate)(w1001, 0.0 ("element"), 0.0 ("element")) -> (w1000:dbl[])
                n336 = Add(x=w1000, y=w1007) -> (x+y=w988:dbl[])
                n337 = Add(x="offset", y=w988) -> (x+y=w987:dbl[])
                "gantry target position" <- w987
                n338 = call "XYZTheta-2Zspeed Go.vi"("error in (no error)"=w1014, "XYZTheta In"=w987, "Motion in"=w1009) -> ("error out"=w1013:errorcluster, "XYZTheta Out"=w1020:dbl[], "Motion out"=w1021:refnum<class "Motion.lvclass">)  [unwired: 6 in]
                n339 = call "1"("error in (no error)"=w1013) -> ("error out"=w1012:errorcluster)  [unwired: 9 in, 1 out]
                n340 = call "Time Delay6"("error in (no error)"=w1012) -> ("error out"=w1011:errorcluster)  [unwired: 10 in]
                n341 = call "WriteReadWait.vi"("Read Value"=w1019, "Write Value"=w1019, "error in (no error)"=w1011, "Read"=w1017, "Write"=w1017, "I-O in"=w1018) -> ("error out"=w991:errorcluster, "I-O out"=w1016:refnum<class "NI-DAQ.lvclass">)  [unwired: 4 in]
                n342 = call "Time Delay4"("error in (no error)"=w991) -> ("error out"=w990:errorcluster)  [unwired: 10 in]
              }
            }
          }
          n343 = call "XYZTheta-2Zspeed Go.vi"("error in (no error)"=w937, "XYZTheta In"=w915, "Motion in"=w944) -> ("error out"=w925:errorcluster, "Motion out"=w948:refnum<class "Motion.lvclass">)  [unwired: 6 in, 1 out]
          n344 = call "Time Delay9"("error in (no error)"=w925) -> ("error out"=w927:errorcluster)  [unwired: 10 in]
          n345 = call-dynamic "Digital Write 1 Channel.vi"("DAQ Module"=0, "error constant"=w927, "Value"=FALSE, "Channel"=0, "NI-DAQ.lvclass"=w930) -> ("error IO"=w926:errorcluster, "NI-DAQ.lvclass 2"=w929:refnum<class "NI-DAQ.lvclass">)  [unwired: 5 in]
          n346 = call "Time Delay10"("error in (no error)"=w926) -> ("error out"=w945:errorcluster)  [unwired: 10 in]
          n347 = call-dynamic "Z Go.vi"("error in (no error)"=w945, "Speed"=10.0, "Position"=0.0 ("new element/subarray"), "Motion in"=w948) -> ("Motion out"=w941:refnum<class "Motion.lvclass">)  [unwired: 6 in, 1 out]
        }
      }
      event "GOTO": Value Change {
        (unwired) "GOING to a position" ("String")
        n348 = event-data() -> ()  [unwired: 1 in, 6 out]
        n349 = call "XYZTheta Go.vi"("XYZTheta In"="Parking position", "Motion in"=w1058) -> ("Motion out"=w1056:refnum<class "Motion.lvclass">)  [unwired: 7 in, 2 out]
      }
      event "READ Position": Value Change {
        n350 = event-data() -> ()  [unwired: 1 in, 6 out]
        n351 = call-dynamic "Get Current Position.vi"("Motion in"=w1077) -> ("XYZTheta Out"=→"Gantry current position":dbl[], "Motion out"=w1076:refnum<class "Motion.lvclass">)  [unwired: 8 in, 1 out]
      }
      event "HDI vacuum": Value Change {
        n352 = event-data() -> ()  [unwired: 1 in, 6 out]
        n353 = call "WriteReadWait.vi"("Read Value"="vacuum", "Write Value"="vacuum", "Read"=w1089, "Write"=w1089, "I-O in"=w1092) -> ("error out"=w1090:errorcluster, "I-O out"=w1079:refnum<class "NI-DAQ.lvclass">)  [unwired: 5 in]
        n354 = call "Time Delay2"("error in (no error)"=w1090) -> ()  [unwired: 10 in, 1 out]
      }
      event Timeout {
        n355 = event-data() -> ()  [unwired: 1 in, 3 out]
        n356 = call-dynamic "Digital Read 1 Channel.vi"("Read"=w1104, "NI-DAQ in"=w1105) -> ("Value"=→"Status":bool, "NI-DAQ out"=w1103:refnum<class "NI-DAQ.lvclass">)  [unwired: 7 in, 1 out]
      }
    }
    "Measured HDI size" <- w25
    "MPT positions on stave" <- w26
    "Stave mark" <- w24
    "measured HDI top-left position" <- w21
    n357 = feedback-in #1(w25) -> ()
    n358 = feedback-in #2(w24) -> ()
    n359 = feedback-in #3(w21) -> ()
    n360 = feedback-in #4(w10) -> ()
    n361 = feedback-in #5(w36) -> ()
    n362 = feedback-in #6(w33) -> ()
    n363 = feedback-in #7(w41) -> ()
    n364 = feedback-in #8(w26) -> ()
    n365 = feedback-in #9(w42) -> ()
    "# of tasks excuted" <- w38
  }
  n366 = call-dynamic "Disconnect.vi"("Controller in"=w4) -> ()  [unwired: 9 in, 1 out]
  n367 = call-dynamic "Disconnect.vi"("I-O in"=w1) -> ()  [unwired: 9 in, 1 out]
